vi "prius_ver0.vi"() -> ()   [LabVIEW 2015]
uses:
  <vilib>/Platform/TimedLoop/XDataNode/timing_clust.ctl
  <vilib>/Platform/TimedLoop/XDataNode/nitl_modes.ctl
  <vilib>/Platform/TimedLoop/XDataNode/wakeup.ctl
  <vilib>/myRIO/Instrument Drivers/Onboard IO/DIO/typedefs/DIO Reference.ctl
  <vilib>/myRIO/Common/Instrument Driver Framework/Utilities/typedefs/myRIO Generic Hardware Reference.ctl
  <vilib>/myRIO/Common/Instrument Driver Framework/Utilities/typedefs/Hardware Version Enum.ctl
  <vilib>/myRIO/Common/Instrument Driver Framework/Utilities/typedefs/myRIO v1.0 Reference.ctl
  <vilib>/myRIO/Common/Instrument Driver Framework/Utilities/typedefs/Generic FPGA Reference.ctl
  <vilib>/myRIO/Common/Instrument Driver Framework/myRIO v1.0/DIO/typedefs/DIO Channels List.ctl
  <vilib>/myRIO/Common/Instrument Driver Framework/myRIO v1.0/DIO/typedefs/DIO Channels Enum.ctl
  <vilib>/userdefined/High Color/nirio_resource_hc.ctl
  <vilib>/myRIO/Common/Instrument Driver Framework/myRIO v1.0/DIO/vis/myRIO v1.1 Open DIO.vi
  <vilib>/myRIO/Common/Instrument Driver Framework/Utilities/vis/Validate Channels.vi
  <vilib>/myRIO/Common/Instrument Driver Framework/myRIO v1.0/DIO/vis/myRIO v1.0 Reserve DIO.vi
  <vilib>/myRIO/Instrument Drivers/Onboard IO/PWM/vis/Set Duty Cycle and Frequency.vi
  <vilib>/myRIO/Common/Instrument Driver Framework/myRIO v1.0/DIO/vis/myRIO v1.0 Close DIO.vi
  <vilib>/myRIO/Common/Instrument Driver Framework/myRIO v1.0/AO/vis/myRIO v1.0 Close AO.vi
  <vilib>/myRIO/Common/Instrument Driver Framework/myRIO v1.0/PWM/vis/myRIO v1.0 Close PWM.vi
  <vilib>/myRIO/Common/Instrument Driver Framework/myRIO v1.0/Resource Manager/vis/myRIO v1.0 Reserve Channel List.vi
  <vilib>/myRIO/Common/Instrument Driver Framework/myRIO v1.0/DIO/vis/myRIO v1.0 Build MUX Configuration DIO.vi
  <vilib>/myRIO/Common/Instrument Driver Framework/myRIO v1.0/DIO/vis/myRIO v1.0 Unreserve DIO.vi
  <vilib>/myRIO/Common/Instrument Driver Framework/myRIO v1.0/AO/vis/myRIO v1.0 Unreserve AO.vi
  <vilib>/myRIO/Common/Instrument Driver Framework/myRIO v1.0/PWM/vis/myRIO v1.0 Unreserve PWM.vi
  <vilib>/myRIO/Common/Instrument Driver Framework/myRIO v1.0/Resource Manager/vis/myRIO v1.0 Reserve Channel.vi
  <vilib>/myRIO/Common/Instrument Driver Framework/myRIO v1.0/Resource Manager/vis/myRIO v1.0 Unreserve Channel.vi
  <vilib>/myRIO/Common/Instrument Driver Framework/myRIO v1.0/Resource Manager/vis/myRIO v1.0 Create Configuration List.vi
  <vilib>/myRIO/Common/Instrument Driver Framework/myRIO v1.0/Resource Manager/vis/myRIO v1.0 Unreserve Channel List.vi
  <vilib>/myRIO/Common/Instrument Driver Framework/myRIO v1.0/AO/vis/myRIO v1.0 Build MUX Configuration AO.vi
  <vilib>/myRIO/Common/Instrument Driver Framework/myRIO v1.0/PWM/vis/myRIO v1.0 Build MUX Configuration PWM.vi
  <vilib>/myRIO/Common/Instrument Driver Framework/myRIO v1.0/Resource Manager/vis/myRIO v1.0 Build Mutex Name.vi
  rio_Global.vi
  <vilib>/Utility/error.llb/Error Cluster From Error Code.vi
  <vilib>/myRIO/Common/Instrument Driver Framework/myRIO v1.0/PWM/vis/myRIO v1.0 Write PWM.vi
  <vilib>/Utility/VariantDataType/GetNumericInfo.vi
  <vilib>/myRIO/Common/Instrument Driver Framework/myRIO v1.0/myRIO v1.1 Open.vi
  <vilib>/myRIO/Common/Instrument Driver Framework/Utilities/vis/IO Manager.vi
  <vilib>/myRIO/Common/Instrument Driver Framework/Utilities/vis/Configuration Manager.vi
  <vilib>/myRIO/Common/Instrument Driver Framework/myRIO v1.0/Resource Manager/vis/myRIO v1.0 Configure IO.vi
  <vilib>/myRIO/Common/Instrument Driver Framework/myRIO v1.0/myRIO v1.0 Close.vi
  <vilib>/myRIO/Common/Instrument Driver Framework/myRIO v1.0/DIO/vis/myRIO v1.0 Write DIO.vi
  <vilib>/myRIO/Common/Instrument Driver Framework/myRIO v1.0/AO/vis/myRIO v1.0 Write AO.vi
  <vilib>/myRIO/Common/Instrument Driver Framework/myRIO v1.0/DIO/vis/myRIO v1.0 Shutdown DIO.vi
  <vilib>/myRIO/Common/Instrument Driver Framework/myRIO v1.0/PWM/vis/myRIO v1.0 Shutdown PWM.vi
  <vilib>/Analysis/Matrix/Numeric/Conversions/Array To Matrix - RA2.vi
  <vilib>/Analysis/Matrix/Numeric/Multiply/Multiply - RM,RM.vi
  <vilib>/Analysis/Matrix/Numeric/Add/Add - RM,RM.vi
  <vilib>/Analysis/baseanly.llb/Real Inverse Matrix.vi
  <vilib>/Analysis/Matrix/Numeric/Subtract/Subtract - RM,RM.vi
  <vilib>/Analysis/Matrix/Numeric/Conversions/Array To Matrix - RA.vi
  <vilib>/Analysis/Matrix/Numeric/Multiply/Multiply - R,RM.vi
  <vilib>/Analysis/Matrix/Numeric/Conversions/Matrix To Array - RM.vi
  <vilib>/myRIO/Instrument Drivers/Onboard IO/DIO/vis/myRIO DIO Open.xnode
  <vilib>/platform/TimedLoop/XDataNode/XDataNode.xnode
  <vilib>/myRIO/Instrument Drivers/Onboard IO/DIO/DIO.lvlib
  <vilib>/myRIO/Instrument Drivers/Onboard IO/PWM/PWM.lvlib
  <vilib>/myRIO/Instrument Drivers/Onboard IO/AO/AO.lvlib
  <vilib>/Analysis/Matrix/NI_Matrix.lvlib
  <vilib>/Analysis/NI_AALBase.lvlib
  <vilib>/Platform/TimedLoop/XDataNode/XDNodeRunTimeDep.lvlib
panel:
  in  "Ref_str_torque":dbl
  in  "invgain>1":dbl=4.499999999999998
  in  "mode":bool=TRUE
  in  "x":dbl
  out "Waveform Chart 2":dynamicdata(graph)=[{"t0"=timestamp(3543844041.358625 s since 1904-01-01), "dt"=1.0, "Y"=[0.015263023114702498]}, {"t0"=timestamp(3543844041.358625 s since 1904-01-01), "dt"=1.0, "Y"=[76.5]}]
  in  "x 2":dbl=0.002000000000000001 format="%#_13g"
  out "Ref_VS":dbl
  in  "y":dbl=0.003
  in  "min vel":i32=20
  in  "shift":dbl
  in  "lpf":dbl=0.8 format="%#_13g"
  in  "gain":dbl=0.79
  in  "str_gain":dbl=0.9 format="%#_13g"
  out "handle":dbl=-0.015263023114702498
  out "lane both":bool=TRUE
  out "get map name":bool
  out "map name":T1(ring)=enum."KAIST"
  in  "Steering Control":bool=TRUE
  out "fake_Ref_speed":dbl
  out "fake_Ref_str_ang":dbl
  out "Waveform Chart":dynamicdata(graph)=[{"t0"=timestamp(3543844041.358625 s since 1904-01-01), "dt"=1.0, "Y"=[0.015263023114702498]}, {"t0"=timestamp(3543844041.358625 s since 1904-01-01), "dt"=1.0, "Y"=[76.5]}]
  out "Gear":u8(ring) items=["P", "R", "N", "D"]
  out "read buffer":string="$GNGGA,114428.80,3623.46520,N,12724.00279,E,2,12,0.81,53.9,M,20.0,M,,0000*7B\r\n"
  out "yaw_rate":dbl=0.25
  out "XY Graph":cluster{"Y":dbl[], "Y":dbl[]}[](graph)=[{"Y"=[1.875, 1.875, 1.875, 1.875, 1.875, 1.875, 1.875, 1.875, 1.875, 1.875], "Y"=[0.0, 0.5, 1.0, 1.5, 2.0, 2.5, 3.0, 3.5, 4.0, 4.5]}, {"Y"=[-1.875, -1.875, -1.875, -1.875, -1.875, -1.875, -1.875, -1.875, -1.875, -1.875], "Y"=[0.0, 0.5, 1.0, 1.5, 2.0, 2.5, 3.0, 3.5, 4.0, 4.5]}, {"Y"=[-0.94, 0.94, 0.94, -0.94, -0.94], "Y"=[-3.2, -3.2, 1.5, 1.5, -3.2]}, {"Y"=[0.0, 0.0, 0.0, 0.0, 0.0, 0.0, 0.0, 0.0, 0.0, 0.0], "Y"=[0.0, 0.5, 1.0, 1.5, 2.0, 2.5, 3.0, 3.5, 4.0, 4.5]}, {"Y"=[-0.0, 0.002441079435136828, 0.009765016068527643, 0.021973905883363898, 0.03907124551911778, 0.061061937284492274, 0.08795229619902045, 0.11975005908698932, 0.15646439575426996, 0.19810592228603952, 0.2446867165104507, 0.2962203356814186, 0.3527218364413329, 0.41420779713322275, 0.48069634254055416, 0.5522071711422214, 0.6287615849803672, 0.7103825222489633, 0.7970945927225799, 0.8889241161567654, 0.9858991638044046, 1.0880496032065068, 1.1954071464308669, 1.3080054019486056, 1.4258799303560679, 1.5490683041691753, 1.677610171938241, 1.811547326954198, 1.950923780842551, 2.095785842368791, 2.246182201809347], "Y"=[0.0, 0.5, 1.0, 1.5, 2.0, 2.5, 3.0, 3.5, 4.0, 4.5, 5.0, 5.5, 6.0, 6.5, 7.0, 7.5, 8.0, 8.5, 9.0, 9.5, 10.0, 10.5, 11.0, 11.5, 12.0, 12.5, 13.0, 13.5, 14.0, 14.5, 15.0]}, {"Y"=[-0.0, 0.0008216505896712079, 0.0032866289850517205, 0.00739501506930651, 0.013146941995614725, 0.020542596208514396, 0.029582217474256822, 0.040266098919687465, 0.05259458707971021, 0.06656808195359076, 0.08218703706990027, 0.09945195956012753, 0.11836341024121566, 0.13892200370679575, 0.16112840842706078, 0.18498334685799023, 0.21048759555890229, 0.23764198531947045, 0.2664474012953235, 0.2969047831529963, 0.32901512522389, 0.3627794766672423, 0.39819894164267566, 0.4352746794916982, 0.474007904928726, 0.5143998882415417, 0.5564519555013874, 0.6001654887822383, 0.6455419263903934, 0.6925827631032746, 0.7412895504183155], "Y"=[0.0, 0.5, 1.0, 1.5, 2.0, 2.5, 3.0, 3.5, 4.0, 4.5, 5.0, 5.5, 6.0, 6.5, 7.0, 7.5, 8.0, 8.5, 9.0, 9.5, 10.0, 10.5, 11.0, 11.5, 12.0, 12.5, 13.0, 13.5, 14.0, 14.5, 15.0]}]
  out "Heading":dbl=-179.220077008385
  out "H_GPS":dbl
  out "pos":dbl[](array[numeric])=[1736.3543614568478, 3514.6262112945274]
  in  "GPS init":bool
  out "pos_gps":dbl[](array[numeric])=[42268800.0, 1.0, 1735.3231710957089, 3511.903145121578, -49.202530661854894, 42268800.0, 12.0, 18.0, 0.0, 0.81, 0.81, 0.0, 36.391086666666666, 127.4000465, 73.0] format="%#_19f"
  out "dt":dbl
  out "ecef ref":dbl[](array[numeric])=[-3119987.903302517, 4086549.99824973, 3761829.662354208]
  out "vgain":dbl=1.0353330715599283
  out "vcount":u64=227
  out "hbias":dbl=0.2579217148182668
  out "hcount":u64=1073
  out "get heading":bool
  out "get position":bool=TRUE
  out "heading error":dbl=3.127980429474107
  out "h_gps":dbl
  out "rt":dbl
  out "pos error":dbl=2.9758035193747063
  out "Kalmann init":bool
  out "VS_CAN":dbl
  out "car":refnum<k5>
  out "mdps str_ang":dbl=76.5
  out "eye":refnum<k5>
  out "APV":dbl
  out "PWM GAS":dbl=1000.0 min=1000.0 max=2000.0 step=1.0
  out "Auto":bool
  in  "Steering angle input":dbl(slide) min=-90.0 max=90.0 step=1.0 scale=-90.0..90.0
  in  "Steering angle input":bool=TRUE
  out "T init":i32=20
  out "T out":i32=20
  in  "manual speed":dbl
  in  "Velocity input":bool
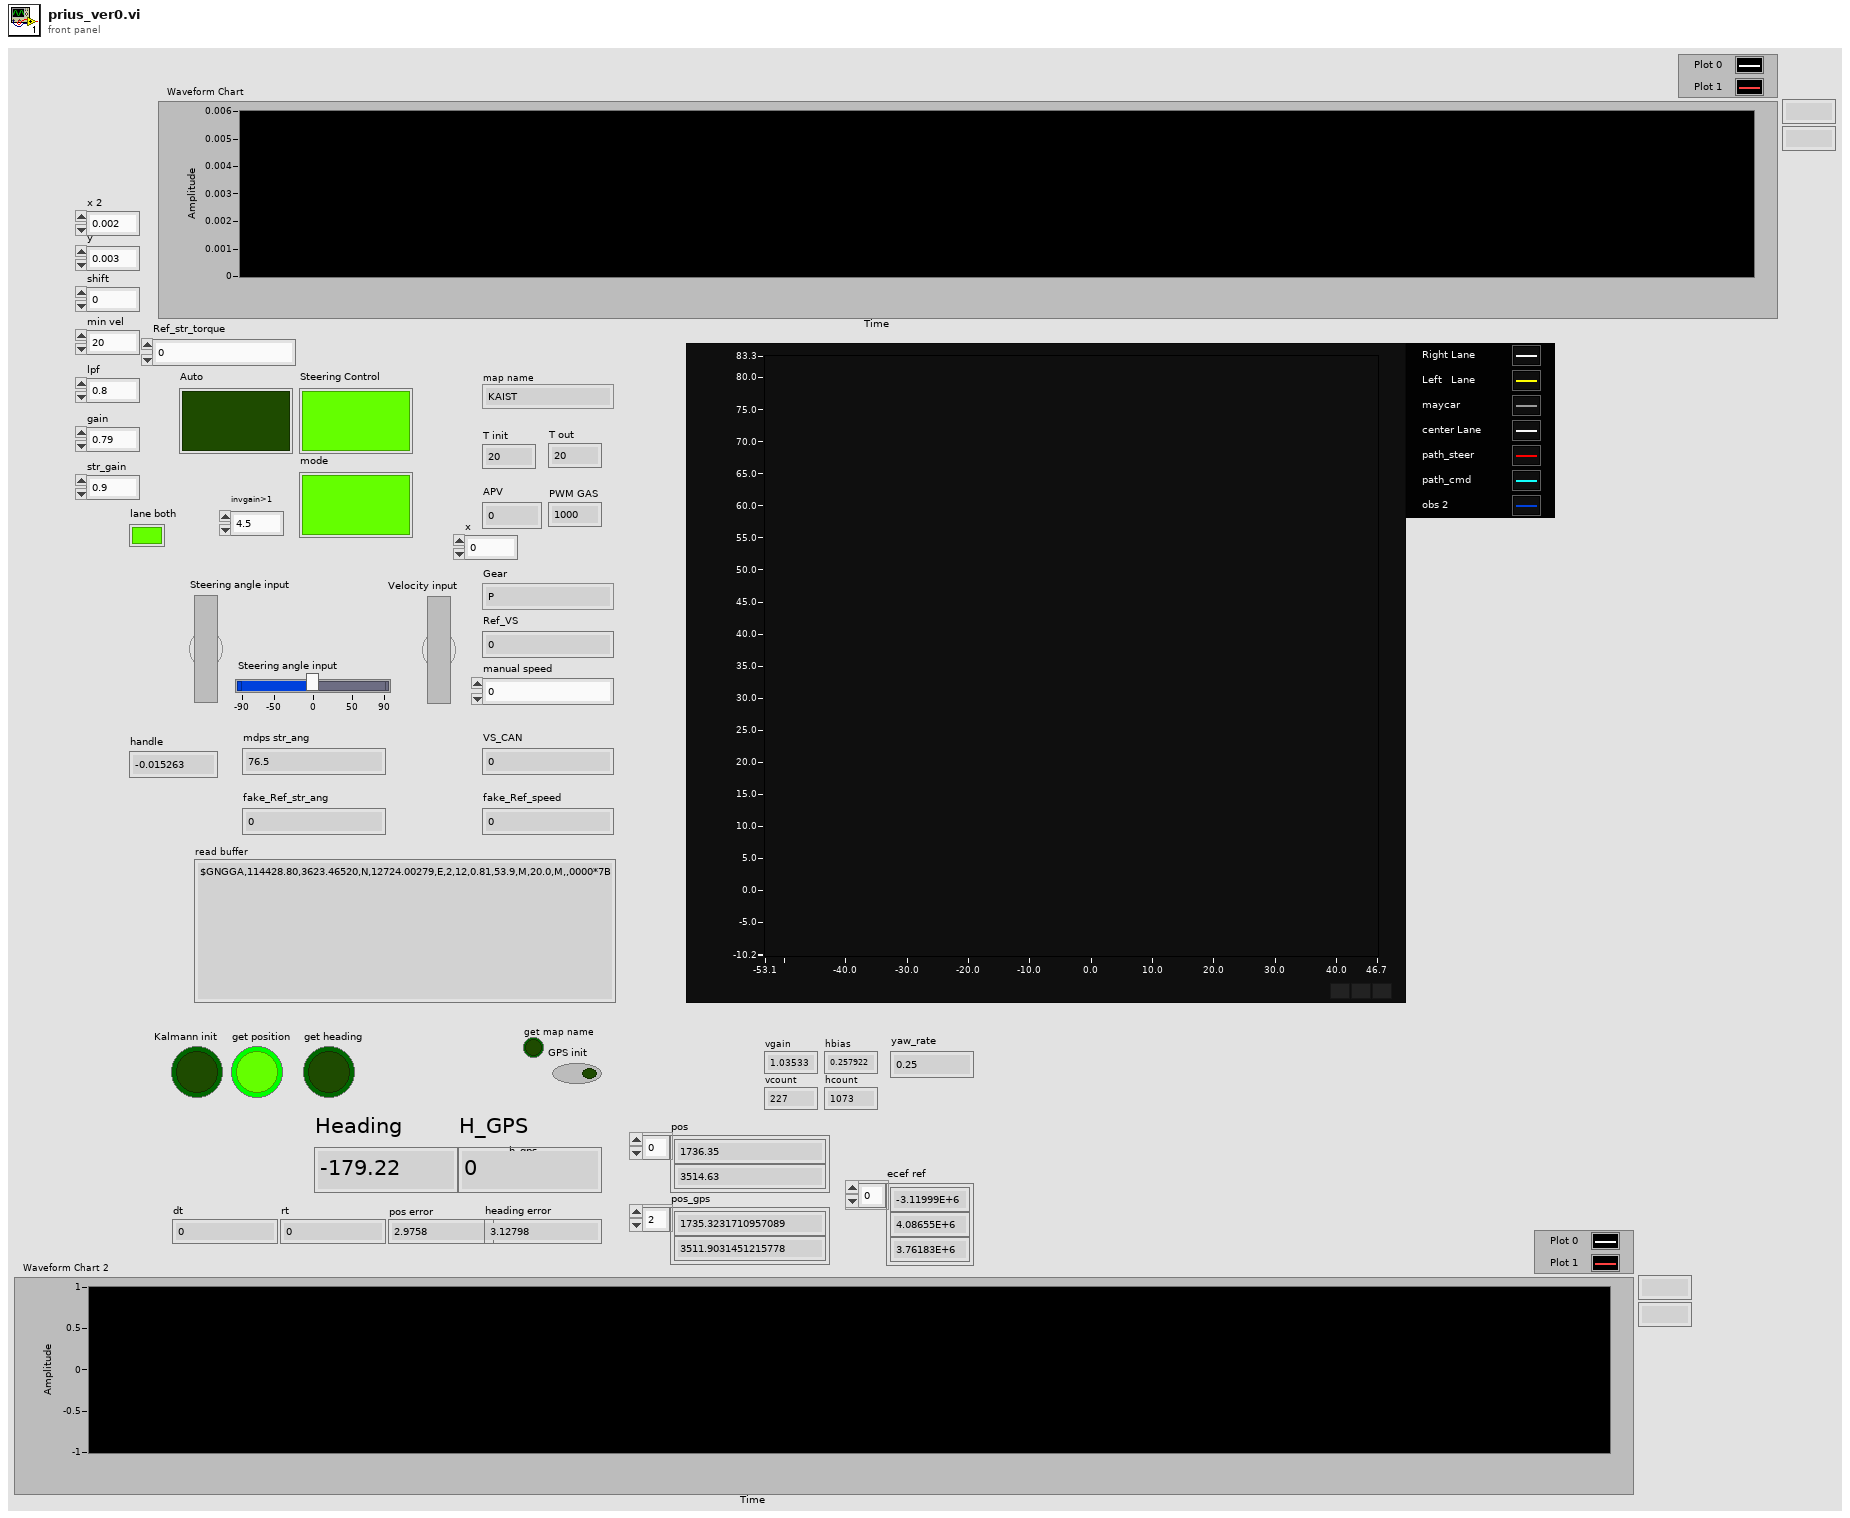
[diagram p1: front panel]
types:
  T1 = enum32{"Namyang", "Hyundai", "KAIST", "Ajou", "Munji", "Airforce", "Car", "KATRI", "Samsung", "Coex", "Gwangnaru"}
  T2 = typedef "XDNodeRunTimeDep.lvlib/timing_clust.ctl" = cluster{"Expected End [f-1]":u64, "Actual End [f-1]":u64, "Finished Late? [f-1]":bool, "Expected End [i-1]":u64, "Actual End [i-1]":u64, "Finished Late? [i-1]":bool, "Expected Start [i]":u64, "Actual Start [i]":u64, "Expected Start [f]":u64, "Actual Start [f]":u64, "Source Name":string, "Structure Name":string, "Period":i64, "Deadline":i64, "Offset":i64, "Start":i64, "Priority":i32, "Timeout":i32, "Mode":T3, "Wakeup Reason":T4, "Error":errorcluster, "Source Type":string, "Secondary Source Type":string, "Global End Time":u64, "Global Start Time":u64, "Frame Duration":u64, "Iteration Duration":u64, "Assigned CPU":i32, "I/O Scan Engine Mode":u32}
  T3 = typedef "XDNodeRunTimeDep.lvlib/nitl_modes.ctl" = enum32{"No Change", "Process missed periods, maintain original phase", "Discard missed periods, maintain original phase", "Process missed periods, ignore original phase", "Discard missed periods, ignore original phase"}
  T4 = typedef "XDNodeRunTimeDep.lvlib/wakeup.ctl" = enum32{"Normal", "Aborted", "Asynchronous wakeup", "Timing source error", "Timed loop error", "Timeout"}
  T5 = typedef "nirio_resource_hc.ctl" = tag
  T6 = typedef "Hardware Version Enum.ctl" = enum16{"Unknown", "myRIO-1900", "myRIO-1950", "roboRIO"}
  T7 = enum16{"Standard", "Buffered", "CRLF", "Immediate"}
  T8 = cluster{"identifier":u32, "timestamp":timestamp, "payload":u8[]}
  T9 = cluster{"connection ID":refnum<k16>, "net address":u32, "port":u16}
  T10 = cluster{"hash":i64, "sys time":i64, "size":i32, "data":u8[]}
  T11 = cluster{"hash":i64, "sys time":i64, "time":dbl, "yaw_rate":dbl, "mdps torque":dbl, "mdps str_ang":dbl, "VS_CAN":dbl, "lat_accel":dbl, "mcp":dbl, "accel pedal value":dbl, "tps":dbl, "odometer":dbl, "battery voltage":dbl, "WHL_SPD_RR":dbl, "WHL_SPD_RL":dbl, "WHL_SPD_FR":dbl, "WHL_SPD_FL":dbl}
  T12 = typedef "PWM.lvlib/PWM Reference.ctl" = cluster{"myRIO Reference":T13, "PWM Channels Enum":T16, "PWM Configuration":T17}
  T13 = typedef "myRIO Generic Hardware Reference.ctl" = cluster{"myRIO Model":T6, "myRIO Hardware Reference":T14}
  T14 = typedef "myRIO v1.0 Reference.ctl" = cluster{"Generic FPGA Reference":T15, "Allow multiple opens":bool}
  T15 = typedef "Generic FPGA Reference.ctl" = refnum<k20>
  T16 = typedef "PWM Channels Enum.ctl" = enum16{"Not Connected", "C/PWM0", "C/PWM1", "A/PWM0", "A/PWM1", "A/PWM2", "B/PWM0", "B/PWM1", "B/PWM2", "PWM/PWM0", "PWM/PWM1", "PWM/PWM2", "PWM/PWM3", "PWM/PWM4", "PWM/PWM5", "PWM/PWM6", "PWM/PWM7", "PWM/PWM8", "PWM/PWM9"}
  T17 = typedef "PWM.lvlib/PWM Configuration.ctl" = cluster{"Frequency":dbl, "Duty Cycle":dbl}
  T18 = typedef "AO.lvlib/AO Reference.ctl" = cluster{"myRIO Reference":T13, "AO Channel List":T19, "AO Scaling Constant List":T21}
  T19 = typedef "AO Channels List.ctl" = T20[]
  T20 = typedef "AO Channels Enum.ctl" = enum16{"Not Connected", "AudioOut/Left", "AudioOut/Right", "C/AO0", "C/AO1", "A/AO0", "A/AO1", "B/AO0", "B/AO1"}
  T21 = typedef "Analog Scaling Constants List.ctl" = T22[]
  T22 = typedef "Analog Scaling Constants.ctl" = cluster{"LSB Weight (Volts)":dbl, "Offset (Volts)":dbl, "Signed?":bool}
  T23 = typedef "DIO.lvlib/DIO Reference.ctl" = cluster{"myRIO Reference":T13, "DIO Channels List":T24}
  T24 = typedef "DIO Channels List.ctl" = T25[]
  T25 = typedef "DIO Channels Enum.ctl" = enum16{"Not Connected", "C/DIO0", "C/DIO1", "C/DIO2", "C/DIO3", "C/DIO4", "C/DIO5", "C/DIO6", "C/DIO7", "A/DIO0", "A/DIO1", "A/DIO2", "A/DIO3", "A/DIO4", "A/DIO5", "A/DIO6", "A/DIO7", "A/DIO8", "A/DIO9", "A/DIO10", "A/DIO11", "A/DIO12", "A/DIO13", "A/DIO14", "A/DIO15", "B/DIO0", "B/DIO1", "B/DIO2", "B/DIO3", "B/DIO4", "B/DIO5", "B/DIO6", "B/DIO7", "B/DIO8", "B/DIO9", "B/DIO10", "B/DIO11", "B/DIO12", "B/DIO13", "B/DIO14", "B/DIO15", "LED0", "LED1", "LED2", "LED3", "Button0", "DIO/DIO0", "DIO/DIO1", "DIO/DIO2", "DIO/DIO3", "DIO/DIO4", "DIO/DIO5", "DIO/DIO6", "DIO/DIO7", "DIO/DIO8", "DIO/DIO9", "SPI/CS0", "SPI/CS1", "SPI/CS2", "SPI/CS3", "LED RADIO (Green)", "LED RADIO (Red)", "LED COMM (Green)", "LED COMM (Red)", "LED MODE (Green)", "LED MODE (Red)"}
  T26 = cluster{"hash":i64, "sys time":i64, "ref_vel":dbl, "ref_steer":dbl, "alert":u8}
  T27 = cluster{"hash":i64, "sys time":i64, "ref_vel":dbl, "ref_steer":dbl}
  T28 = cluster{"hash":i64, "sys time":i64, "Auto":bool, "Run":bool, "Solenoid":bool, "T lim":bool, "brk_enc":u8, "B PWM":u16, "T PWM":u16, "ref_vel":dbl, "ref_bkr_enc":dbl, "ref_apv":dbl, "ref_steer":dbl}
  T29 = typedef "NI_Matrix.lvlib/RealMatrix.ctl" = dbl[][]
  T30 = cluster{"hash":i64, "sys time":i64, "dt":dbl, "x":dbl, "y":dbl, "speed":dbl, "heading":dbl, "yaw_rate":dbl}
  T31 = cluster{"Real 2D Array[0]":dbl, "Real 2D Array[1]":dbl, "Real 2D Array[2]":dbl, "Real 2D Array[3]":dbl, "Real 2D Array[4]":dbl}
  T32 = cluster{"hash":i64, "sys time":i64, "time":dbl, "x":dbl, "y":dbl, "h":dbl, "numSV":i32, "postype":i32, "lag":i32, "hordev":dbl, "lat":dbl, "lon":dbl, "hgt":dbl, "map_idx":i32}
  T33 = cluster{"output[0]":dbl, "output[1]":dbl, "output[2]":dbl, "output[3]":dbl, "output[4]":dbl, "output[5]":dbl, "output[6]":dbl, "output[7]":dbl, "output[8]":dbl, "output[9]":dbl, "output[10]":dbl, "output[11]":dbl, "output[12]":dbl, "output[13]":dbl, "output[14]":dbl}
  T34 = cluster{"hash":i64, "sys time":i64, "time":dbl, "speed":dbl, "heading":dbl, "lat":dbl, "lon":dbl}
  T35 = cluster{"output[0]":dbl, "output[1]":dbl, "output[2]":dbl, "output[3]":dbl, "output[4]":dbl, "output[5]":dbl, "output[6]":dbl}
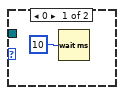
[diagram p2: hidden frame]
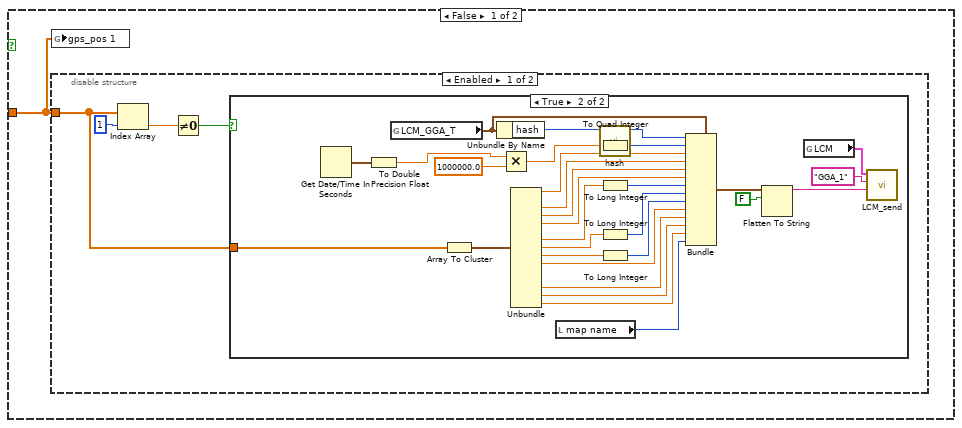
[diagram p4: hidden frame]
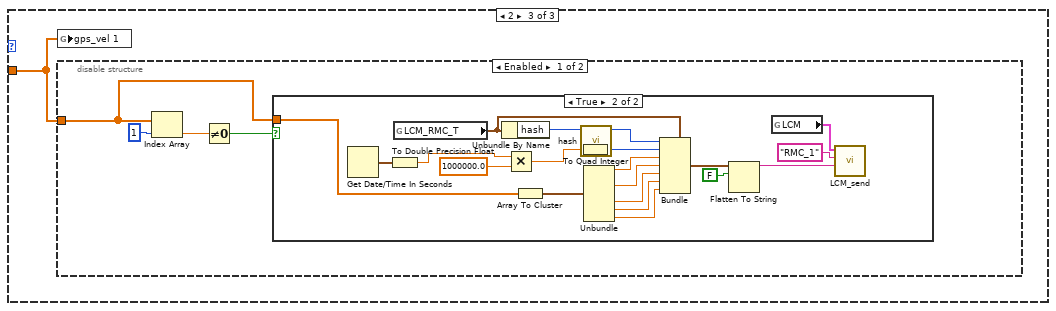
[diagram p7: hidden frame]
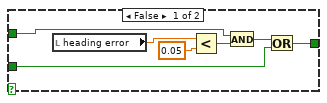
[diagram p13: hidden frame]
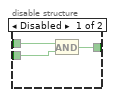
[diagram p14: hidden frame]
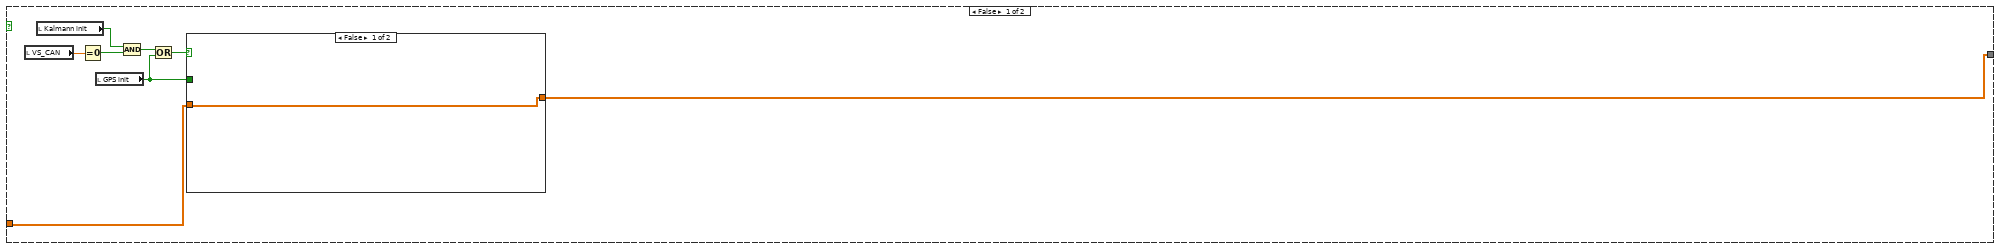
[diagram p15: hidden frame]
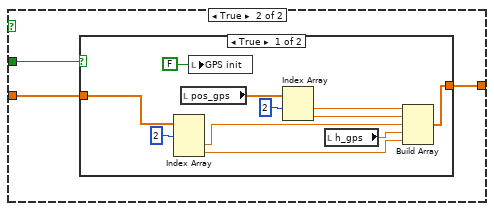
[diagram p16: hidden frame]
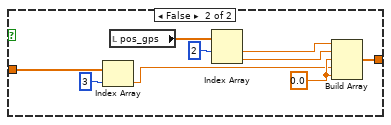
[diagram p17: hidden frame]
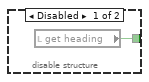
[diagram p19: hidden frame]
diagram:
  n1 = flat-sequence {
    frame #0 {
      w17 = u16 7668 ("port")
      w13 = u16 7665 ("port")
      n2 = disable-structure shown="Enabled" {
        frame Disabled {
        }
        frame Enabled {
          w36 = "Prius" ("Car_name")
          w37 = 0.0 ("Ref_str_ang")
          w38 = 1000.0 ("PWM GAS")
          w34 = FALSE ("Auto SW")
          n3 = global write "rio_Global.vi" "steering torque"(0.0 ("steering")) -> ()
          n4 = global write "rio_Global.vi" "Shift control"(0.0 ("Shift control")) -> ()
          n5 = global write "rio_Global.vi" "Solenoid"(FALSE ("CAN A 1")) -> ()
          n6 = global write "rio_Global.vi" "PWM GAS"(w38) -> ()
          n7 = global write "rio_Global.vi" "PWM Brake"(w38) -> ()
          n8 = global write "rio_Global.vi" "Ref_VS"(w37) -> ()
          n9 = global write "rio_Global.vi" "Ref_str_ang"(w37) -> ()
          n10 = global write "rio_Global.vi" "Auto"(w34) -> ()
          n11 = global write "rio_Global.vi" "Car_name"(w36) -> ()
          n12 = call "car_spec.vi"("Car_name"=w36) -> ("wheel base"=w31:dbl, "ratio"=w32:dbl, "overall width"=w33:dbl)  [unwired: 5 in, 3 out]
          n13 = global write "rio_Global.vi" "Auto SW"(w34) -> ()
          n14 = global write "rio_Global.vi" "ratio"(w32) -> ()
          n15 = global write "rio_Global.vi" "overall width"(w33) -> ()
          n16 = global write "rio_Global.vi" "wheel base"(w31) -> ()
        }
      }
      n17 = local read "eye"() -> (w19:refnum<k5>)
      n18 = local read "car"() -> (w20:refnum<k5>)
      n19 = global read "rio_Global.vi" "LCM PC"() -> (w10:T9)
      n20 = Equal?(x=refnum<k5> refnum ("connection ID"), y=w19) -> (x = y?=w21:bool)
      n21 = Equal?(x=refnum<k5> refnum ("connection ID"), y=w20) -> (x = y?=w23:bool)
      n22 = UDP Open(11:w17) -> (port=w15:refnum<k16>)  [unwired: 4 in, 2 out]
      n23 = Decrement(x=w13) -> (x-1=w12:u16)
      n24 = disable-structure shown="Enabled" {
        disable-tunnel: [w26 w29] -> w14
        disable-tunnel: w12 -> [w25 w30]
        frame Enabled {
          n25 = UDP Open(11:w25) -> (port=w26:refnum<k16>)  [unwired: 4 in, 2 out]
        }
        frame Disabled {
          n26 = String To IP(1:"239.255.76.67" ("name")) -> (0:w27:u32)
          n27 = UDP Multicast Open(10:w27, 11:w30) -> (3:w29:refnum<k16>)  [unwired: 3 in, 2 out]
        }
      }
      n28 = case shown="False" w21 {
        tunnel: w19 -> [w42 _]
        tunnel: [w41 w47] -> w18
        frame False {
          n29 = flat-sequence {
            tunnel: w42 -> [w43]
            tunnel: [w44] -> w41
            frame #0 {
              n30 = TCP Close Connection(connection ID=w43) -> ()  [unwired: 2 in, 2 out]
            }
            frame #1 {
              w45 = u16 3000  # port
              n31 = TCP Open Connection(address="192.168.0.100", remote port or service name=w45) -> (connection ID=w44:refnum<k5>)  [unwired: 3 in, 1 out]
            }
          }
        }
        frame True {
          w48 = u16 3000  # port
          n32 = TCP Open Connection(address="192.168.0.100", remote port or service name=w48) -> (connection ID=w47:refnum<k5>)  [unwired: 3 in, 1 out]
        }
      }
      "eye" <- w18
      n33 = case shown="False" w23 {
        tunnel: w20 -> [w51 _]
        tunnel: [w50 w56] -> w5
        frame False {
          n34 = flat-sequence {
            tunnel: w51 -> [w52]
            tunnel: [w53] -> w50
            frame #0 {
              n35 = TCP Close Connection(connection ID=w52) -> ()  [unwired: 2 in, 2 out]
            }
            frame #1 {
              w54 = u16 4000  # port
              n36 = TCP Open Connection(address="192.168.0.200", remote port or service name=w54) -> (connection ID=w53:refnum<k5>)  [unwired: 3 in, 1 out]
            }
          }
        }
        frame True {
          w57 = u16 4000  # port
          n37 = TCP Open Connection(address="192.168.0.200", remote port or service name=w57) -> (connection ID=w56:refnum<k5>)  [unwired: 3 in, 1 out]
        }
      }
      n38 = Bundle By Name(cluster=w10, "port"=w17, "connection ID"=w15, "net address"=u32 0) -> (w11:T9)
      n39 = global write "rio_Global.vi" "LCM PC"(w11) -> ()
      n40 = String To IP(1:"192.168.0.5" ("name")) -> (0:w2:u32)
      n41 = global read "rio_Global.vi" "LCM"() -> (w9:T9)
      n42 = Bundle By Name(cluster=w9, "port"=w13, "connection ID"=w14, "net address"=w2) -> (w8:T9)
      n43 = global write "rio_Global.vi" "LCM"(w8) -> ()
      n44 = TCP Read(connection ID=w5, bytes to read=999999, 9:1 ("timeout ms (25000)")) -> (connection ID out=→"car":refnum<k5>)  [unwired: 2 in, 2 out]
    }
    frame #1 {
      w87 = tag "B/PWM2"  # Brake
      w101 = tag[] ["B/AO0", "B/AO1"]  # Steering
      w108 = tag[] ["B/DIO4"]  # auto
      w111 = tag "B/PWM0"  # Accel
      w116 = tag[] ["B/DIO5", "B/DIO6"]  # Solenoid
      w78 = tag[] ["C/DIO7", "C/DIO6", "C/DIO5", "C/DIO0"]  # Shift X Eable
      w83 = tag[] ["C/AO0", "C/AO1"]  # Shift
      n45 = local read "eye"() -> (w92:refnum<k5>)
      n46 = local read "car"() -> (w88:refnum<k5>)
      n47 = while {
        tunnel: w92 -> [w302]
        tunnel: [w304] -> w95
        tunnel: [w303] -> w94
        shift-right: [w298] -> _
        shift-left: "" -> [w301]
        stop <- FALSE stop-if-true
        n48 = TCP Read(connection ID=w302, bytes to read=999999, 7:T7."Immediate" ("mode (standard)"), 9:1 ("timeout ms (25000)")) -> (connection ID out=w304:refnum<k5>, data out=w300:string, error out=w303:errorcluster)  [unwired: 1 in]
        n49 = Concatenate Strings(w301, w300) -> (w299:string)
        n50 = case shown="Default" w299 {
          selector: w299 -> [_ w312]
          tunnel: [_ w311] -> w298
          frame "" {
          }
          frame Default {
            n51 = flat-sequence {
              tunnel: w312 -> [w313]
              tunnel: [w314] -> w310
              tunnel: [w313] -> w309
              tunnel: [w343] -> w311
              tunnel: w310 -> [w343]
              tunnel: w309 -> [w342]
              frame #0 {
                n52 = while {
                  shift-right: [w321] -> w314
                  shift-left: w313 -> [w333]
                  stop <- w318 stop-if-true
                  w319 = "S" ("regular expression")
                  n53 = Match Pattern(string=w333, regular expression="S") -> (after substring=w331:string)  [unwired: 1 in, 3 out]
                  n54 = Match Pattern(string=w331, regular expression=" ") -> (before substring=w329:string, after substring=w326:string)  [unwired: 1 in, 2 out]
                  n55 = Hexadecimal String To Number(string=w329) -> (number=w316:u32)  [unwired: 2 in, 1 out]
                  n56 = Match Pattern(string=w326, regular expression=w319) -> (before substring=w325:string, match substring=w320:string, after substring=w322:string)  [unwired: 1 in, 1 out]
                  n57 = Not Equal?(x=w320, y=w319) -> (x != y?=w318:bool)
                  n58 = Concatenate Strings(w320, w322) -> (w321:string)
                  n59 = for {
                    N: 8 -> [_]
                    tunnel: w325 -> [w341]
                    tunnel: [w337] -> w315 mode=indexing
                    i -> [w336]
                    n60 = Multiply(x=2, y=w336) -> (x*y=w339:i32)
                    n61 = String Subset(string=w341, offset (0)=w339, length (rest)=2 ("length (rest)")) -> (substring=w334:string)
                    n62 = Hexadecimal String To Number(string=w334, default (0uL)=u8 0) -> (number=w337:u8)  [unwired: 1 in, 1 out]
                  }
                  n63 = Get Date/Time In Seconds() -> (seconds since 1Jan1904=w324:timestamp)
                  n64 = Bundle By Name(cluster=T8 {"identifier"=0, "timestamp"=timestamp(0 s since 1904-01-01), "payload"=[]} ("can cluster"), "identifier"=w316, "payload"=w315, "timestamp"=w324) -> (w323:T8)
                  n65 = call "mobileye_decoder.vi"("can cluster"=w323, "name"="Mobileye560") -> ()  [unwired: 10 in]
                }
              }
              frame #1 {
                n66 = disable-structure shown="Enabled" {
                  disable-tunnel: w342 -> [w345 _]
                  frame Enabled {
                    n67 = global read "rio_Global.vi" "LCM_CAN_RAW_SNAP"() -> (w358:T10)
                    n68 = Get Date/Time In Seconds() -> (seconds since 1Jan1904=w356:timestamp)
                    n69 = To Double Precision Float(number=w356) -> (double precision float=w355:dbl)
                    n70 = Unbundle By Name(w358) -> ("hash"=w353:i64)
                    n71 = Multiply(x=w355, y=1000000.0) -> (x*y=w357:dbl)
                    n72 = String To Byte Array(string=w345) -> (unsigned byte array=w346:u8[])
                    n73 = To Quad Integer(1:w357) -> (0:w348:i64)
                    n74 = call "hash.vi"("input"=w353) -> ("output"=w359:i64)  [unwired: 10 in]
                    n75 = Array Size(array=w346) -> (size(s)=w347:i32)
                    n76 = Bundle(cluster=w358, "hash"=w359, "sys time"=w348, "size"=w347, "data"=w346) -> (w351:T10)
                    n77 = Flatten To String(anything=w351, prepend array or string size? (T)=FALSE) -> (data string=w349:string)  [unwired: 2 in, 2 out]
                    n78 = global read "rio_Global.vi" "LCM"() -> (w350:T9)
                    n79 = call "LCM_send.vi"("DATA"=w349, "ID"="Mobileye560S", "LCM"=w350) -> ()  [unwired: 7 in, 2 out]
                  }
                  frame Disabled {
                  }
                }
              }
            }
          }
        }
      }
      n80 = while {
        tunnel: w88 -> [w209]
        tunnel: [w211] -> w89
        tunnel: [w210] -> w90
        shift-right: [w205] -> _
        shift-left: "" -> [w208]
        stop <- FALSE stop-if-true
        n81 = TCP Read(connection ID=w209, bytes to read=999999, 7:T7."Immediate" ("mode (standard)"), 9:1 ("timeout ms (25000)")) -> (connection ID out=w211:refnum<k5>, data out=w207:string, error out=w210:errorcluster)  [unwired: 1 in]
        n82 = Concatenate Strings(w208, w207) -> (w206:string)
        n83 = case shown="Default" w206 {
          selector: w206 -> [_ w219]
          tunnel: [_ w220] -> w205
          frame "" {
          }
          frame Default {
            n84 = flat-sequence {
              tunnel: w219 -> [w221]
              tunnel: [w222] -> w218
              tunnel: [w221] -> w217
              tunnel: w218 -> [w251]
              tunnel: w217 -> [w250]
              tunnel: [w251] -> w216
              tunnel: [w297] -> w220
              tunnel: w216 -> [w297]
              frame #0 {
                n85 = while {
                  shift-right: [w231] -> w222
                  shift-left: w221 -> [w241]
                  stop <- w228 stop-if-true
                  w229 = "S" ("regular expression")
                  n86 = Match Pattern(string=w241, regular expression="S") -> (after substring=w239:string)  [unwired: 1 in, 3 out]
                  n87 = Match Pattern(string=w239, regular expression=" ") -> (before substring=w237:string, after substring=w235:string)  [unwired: 1 in, 2 out]
                  n88 = Hexadecimal String To Number(string=w237) -> (number=w226:u32)  [unwired: 2 in, 1 out]
                  n89 = Match Pattern(string=w235, regular expression=w229) -> (before substring=w234:string, match substring=w230:string, after substring=w232:string)  [unwired: 1 in, 1 out]
                  n90 = Not Equal?(x=w230, y=w229) -> (x != y?=w228:bool)
                  n91 = Concatenate Strings(w230, w232) -> (w231:string)
                  n92 = for {
                    N: 8 -> [_]
                    tunnel: w234 -> [w249]
                    tunnel: [w245] -> w225 mode=indexing
                    i -> [w244]
                    n93 = Multiply(x=2, y=w244) -> (x*y=w247:i32)
                    n94 = String Subset(string=w249, offset (0)=w247, length (rest)=2 ("length (rest)")) -> (substring=w242:string)
                    n95 = Hexadecimal String To Number(string=w242, default (0uL)=u8 0) -> (number=w245:u8)  [unwired: 1 in, 1 out]
                  }
                  n96 = Get Date/Time In Seconds() -> (seconds since 1Jan1904=w233:timestamp)
                  n97 = Bundle By Name(cluster=T8 {"identifier"=0, "timestamp"=timestamp(0 s since 1904-01-01), "payload"=[]} ("can cluster"), "identifier"=w226, "payload"=w225, "timestamp"=w233) -> (w223:T8)
                  n98 = global read "rio_Global.vi" "Car_name"() -> (w224:string)
                  n99 = call "can decoder.vi"("can cluster"=w223, "name"=w224) -> ()  [unwired: 10 in]
                }
              }
              frame #1 {
                n100 = disable-structure shown="Enabled" {
                  disable-tunnel: w250 -> [w252 _]
                  frame Enabled {
                    n101 = global read "rio_Global.vi" "LCM_CAN_RAW_SNAP"() -> (w254:T10)
                    n102 = Get Date/Time In Seconds() -> (seconds since 1Jan1904=w256:timestamp)
                    n103 = To Double Precision Float(number=w256) -> (double precision float=w257:dbl)
                    n104 = Unbundle By Name(w254) -> ("hash"=w259:i64)
                    n105 = Multiply(x=w257, y=1000000.0) -> (x*y=w255:dbl)
                    n106 = String To Byte Array(string=w252) -> (unsigned byte array=w267:u8[])
                    n107 = To Quad Integer(1:w255) -> (0:w265:i64)
                    n108 = call "hash.vi"("input"=w259) -> ("output"=w253:i64)  [unwired: 10 in]
                    n109 = Array Size(array=w267) -> (size(s)=w266:i32)
                    n110 = Bundle(cluster=w254, "hash"=w253, "sys time"=w265, "size"=w266, "data"=w267) -> (w261:T10)
                    n111 = global read "rio_Global.vi" "Car_name"() -> (w264:string)
                    n112 = Flatten To String(anything=w261, prepend array or string size? (T)=FALSE) -> (data string=w263:string)  [unwired: 2 in, 2 out]
                    n113 = global read "rio_Global.vi" "LCM"() -> (w262:T9)
                    n114 = call "LCM_send.vi"("DATA"=w263, "ID"=w264, "LCM"=w262) -> ()  [unwired: 7 in, 2 out]
                  }
                  frame Disabled {
                  }
                }
              }
              frame #2 {
                n115 = Get Date/Time In Seconds() -> (seconds since 1Jan1904=w288:timestamp)
                n116 = global read "rio_Global.vi" "LCM_CAN_T"() -> (w270:T11)
                n117 = To Double Precision Float(number=w288) -> (double precision float=w289:dbl)
                n118 = global read "rio_Global.vi" "C_mdps str_ang"() -> (w269:dbl)
                n119 = global read "rio_Global.vi" "C_battery voltage"() -> (w273:dbl)
                n120 = global read "rio_Global.vi" "C_WHL_SPD_RR"() -> (w274:dbl)
                n121 = global read "rio_Global.vi" "C_WHL_SPD_RL"() -> (w275:dbl)
                n122 = global read "rio_Global.vi" "C_WHL_SPD_FR"() -> (w271:dbl)
                n123 = global read "rio_Global.vi" "C_WHL_SPD_FL"() -> (w276:dbl)
                n124 = global read "rio_Global.vi" "C_mdps torque"() -> (w283:dbl)
                n125 = Unbundle By Name(w270) -> ("hash"=w291:i64)
                n126 = Multiply(x=w289, y=1000000.0) -> (x*y=w287:dbl)
                n127 = global read "rio_Global.vi" "C_odometer"() -> (w277:dbl)
                n128 = global read "rio_Global.vi" "C_yaw_rate"() -> (w284:dbl)
                n129 = global read "rio_Global.vi" "C_VS_CAN"() -> (w282:dbl)
                n130 = global read "rio_Global.vi" "C_MCP"() -> (w280:dbl)
                n131 = global read "rio_Global.vi" "C_APV"() -> (w279:dbl)
                n132 = To Quad Integer(1:w287) -> (0:w296:i64)
                n133 = Negate(x=w269) -> (-x=w268:dbl)
                n134 = call "hash.vi"("input"=w291) -> ("output"=w286:i64)  [unwired: 10 in]
                n135 = global read "rio_Global.vi" "time"() -> (w285:dbl)
                n136 = Bundle(cluster=w270, "hash"=w286, "sys time"=w296, "time"=w285, "yaw_rate"=w284, "mdps torque"=w283, "mdps str_ang"=w268, "VS_CAN"=w282, "lat_accel"=0.0, "mcp"=w280, "accel pedal value"=w279, "tps"=0.0, "odometer"=w277, "battery voltage"=w273, "WHL_SPD_RR"=w274, "WHL_SPD_RL"=w275, "WHL_SPD_FR"=w271, "WHL_SPD_FL"=w276) -> (w293:T11)
                n137 = Flatten To String(anything=w293, prepend array or string size? (T)=FALSE) -> (data string=w295:string)  [unwired: 2 in, 2 out]
                n138 = global read "rio_Global.vi" "LCM"() -> (w294:T9)
                n139 = call "LCM_send.vi"("DATA"=w295, "ID"="CAN_T", "LCM"=w294) -> ()  [unwired: 7 in, 2 out]
              }
            }
          }
        }
      }
      n140 = call <vilib>:"Smart Open.vi"("Allow multiple opens?"=FALSE, "Channel Name"=w87) -> ("error out"=w61:errorcluster, "PWM Ref Out"=w64:T12)  [unwired: 8 in]
      n141 = call <vilib>:"Smart Open.vi"("Allow multiple opens?"=FALSE, "Channel Name"=w111) -> ("error out"=w69:errorcluster, "PWM Ref Out"=w68:T12)  [unwired: 8 in]
      n142 = call <vilib>:"Set Frequency.vi"("error in (no error)"=w61, "Frequency [Hz]"=50.0, "PWM Ref In"=w64) -> ("error out"=w60:errorcluster, "PWM Ref Out"=w63:T12)  [unwired: 6 in]
      n143 = call <vilib>:"Set Frequency.vi"("error in (no error)"=w69, "Frequency [Hz]"=50.0, "PWM Ref In"=w68) -> ("error out"=w66:errorcluster, "PWM Ref Out"=w67:T12)  [unwired: 6 in]
      n144 = call <vilib>:"Smart Open.vi"("Allow multiple opens?"=TRUE, "Channel Names"=w101) -> ("error out"=w99:errorcluster, "AO Ref Out"=w100:T18)  [unwired: 8 in]
      n145 = call <vilib>:"Smart Open.vi"("Allow multiple opens?"=FALSE, "Channel Names"=w108) -> ("error out"=w106:errorcluster, "DIO Ref Out"=w107:T23)  [unwired: 8 in]
      n146 = xnode "myRIO DIO Open.xnode"("Allow multiple opens?"=TRUE, "Channel Names"=w116) -> ("error out"=w114:errorcluster, "DIO Ref Out"=w115:T23)  [unwired: 1 in]
      n147 = xnode "myRIO DIO Open.xnode"("Allow multiple opens?"=TRUE, "Channel Names"=w78) -> ("error out"=w73:errorcluster, "DIO Ref Out"=w76:T23)  [unwired: 1 in]
      n148 = call <vilib>:"Smart Open.vi"("Allow multiple opens?"=TRUE, "Channel Names"=w83) -> ("error out"=w79:errorcluster, "AO Ref Out"=w82:T18)  [unwired: 8 in]
      n149 = node-c288(i64 10 ("Period")) -> (w72:T2)  [unwired: 3 in]
      n150 = timed-loop {
        tunnel: w115 -> [w181]
        tunnel: [w182] -> w113
        tunnel: w114 -> [w180]
        tunnel: [w176] -> w112
        tunnel: w107 -> [w174]
        tunnel: [w174] -> w105
        tunnel: w106 -> [w173]
        tunnel: [w173] -> w104
        tunnel: w100 -> [w172]
        tunnel: [w170] -> w98
        tunnel: w99 -> [w171]
        tunnel: [w169] -> w97
        tunnel: w67 -> [w178]
        tunnel: [w179] -> w110
        tunnel: w66 -> [w177]
        tunnel: [w175] -> w109
        tunnel: w63 -> [w167]
        tunnel: [w166] -> w85
        tunnel: w82 -> [w165]
        tunnel: [w164] -> w81
        tunnel: [w163] -> w80
        tunnel: w79 -> [w162]
        tunnel: w76 -> [w161]
        tunnel: [w160] -> w75
        tunnel: [w159] -> w74
        tunnel: w73 -> [w158]
        timing: w72 -> [_]
        timing-out: [_] -> w71
        tunnel: w60 -> [w128]
        tunnel: [w127] -> w59
        stop <- FALSE ("Auto") stop-if-true
        w148 = 0.0 ("y")
        n151 = node-c288() -> ()  [unwired: 1 in]
        n152 = global read "rio_Global.vi" "PWM Brake"() -> (w120:dbl)
        n153 = global read "rio_Global.vi" "PWM GAS"() -> (w123:dbl)
        n154 = global read "rio_Global.vi" "Solenoid"() -> (w121:bool)
        n155 = global read "rio_Global.vi" "steering torque"() -> (w144:dbl)
        n156 = global read "rio_Global.vi" "Shift control"() -> (w132:dbl)
        n157 = global read "rio_Global.vi" "C_VS_CAN"() -> (w140:dbl)
        n158 = global read "rio_Global.vi" "Auto"() -> (w119:bool)
        n159 = global read "rio_Global.vi" "Auto"() -> (w124:bool)
        n160 = global read "rio_Global.vi" "Auto"() -> (w122:bool)
        n161 = Select(t=w121, s=w122, f=w122) -> (s? t:f=w126:bool)
        n162 = Negate(x=w144) -> (-x=w146:dbl)
        n163 = Equal To 0?(x=w140) -> (x = 0?=w130:bool)
        n164 = Not Equal To 0?(x=w132) -> (x != 0?=w131:bool)
        n165 = Select(t=w120, s=w119, f=1000.0) -> (s? t:f=w142:dbl)
        n166 = Select(t=w123, s=w124, f=1000.0) -> (s? t:f=w147:dbl)
        n167 = global read "rio_Global.vi" "Auto"() -> (w145:bool)
        n168 = global read "rio_Global.vi" "Auto"() -> (w141:bool)
        n169 = Build Array(w126, w126) -> (w152:bool[])
        n170 = Select(t=w146, s=w145, f=w148) -> (s? t:f=w149:dbl)
        n171 = call <vilib>:"Write.vi"("error in (no error)"=w180, "Values"=w152, "DIO Ref In"=w181) -> ("error out"=w176:errorcluster, "DIO Ref Out"=w182:T23)  [unwired: 6 in]
        n172 = Compound Arithmetic op=AND(w130, w141, w131) -> (w137:bool)
        n173 = Divide(x=w142, y=20000.0) -> (x/y=w129:dbl)
        n174 = Divide(x=w147, y=20000.0) -> (x/y=w150:dbl)
        n175 = Max & Min(x=w149, y=w148) -> (min(x,y)=w154:dbl)  [unwired: 1 out]
        n176 = Select(t=w132, s=w137, f=0.0 ("element")) -> (s? t:f=w134:dbl)
        n177 = Build Array(w137, w137, w137, FALSE ("element")) -> (w139:bool[])
        n178 = call <vilib>:"Write.vi"("error in (no error)"=w158, "Values"=w139, "DIO Ref In"=w161) -> ("error out"=w159:errorcluster, "DIO Ref Out"=w160:T23)  [unwired: 6 in]
        n179 = Negate(x=w154) -> (-x=w153:dbl)
        n180 = call <vilib>:"Set Duty Cycle.vi"("error in (no error)"=w128, "Duty Cycle"=w129, "PWM Ref In"=w167) -> ("error out"=w127:errorcluster, "PWM Ref Out"=w166:T12)  [unwired: 6 in]
        n181 = call <vilib>:"Set Duty Cycle.vi"("error in (no error)"=w177, "Duty Cycle"=w150, "PWM Ref In"=w178) -> ("error out"=w175:errorcluster, "PWM Ref Out"=w179:T12)  [unwired: 6 in]
        n182 = Max & Min(x=0.0, y=w149) -> (max(x,y)=w155:dbl)  [unwired: 1 out]
        n183 = Build Array(0.0 ("element"), w134) -> (w133:dbl[])
        n184 = call <vilib>:"Write.vi"("error in (no error)"=w162, "Values"=w133, "AO Ref In"=w165) -> ("error out"=w163:errorcluster, "AO Ref Out"=w164:T18)  [unwired: 6 in]
        n185 = Build Array(w155, w153) -> (w157:dbl[])
        n186 = call <vilib>:"Write.vi"("error in (no error)"=w171, "Values"=w157, "AO Ref In"=w172) -> ("error out"=w169:errorcluster, "AO Ref Out"=w170:T18)  [unwired: 6 in]
        n187 = node-c288() -> ()  [unwired: 1 out]
      }
      n188 = node-c288(w71) -> ()  [unwired: 1 out]
      n189 = call <vilib>:"Close.vi"("error in (no error)"=w97, "AO Ref In"=w98) -> ()  [unwired: 9 in, 1 out]
      n190 = call <vilib>:"Close.vi"("error in (no error)"=w59, "PWM Ref In"=w85) -> ()  [unwired: 9 in, 1 out]
      n191 = call <vilib>:"Close.vi"("error in (no error)"=w104, "DIO Ref In"=w105) -> ()  [unwired: 9 in, 1 out]
      n192 = call <vilib>:"Close.vi"("error in (no error)"=w109, "PWM Ref In"=w110) -> ()  [unwired: 9 in, 1 out]
      n193 = call <vilib>:"Close.vi"("error in (no error)"=w112, "DIO Ref In"=w113) -> ()  [unwired: 9 in, 1 out]
      n194 = call <vilib>:"Close.vi"("error in (no error)"=w74, "DIO Ref In"=w75) -> ()  [unwired: 9 in, 1 out]
      n195 = call <vilib>:"Close.vi"("error in (no error)"=w80, "AO Ref In"=w81) -> ()  [unwired: 9 in, 1 out]
      n196 = TCP Close Connection(connection ID=w95, error in (no error)=w94) -> ()  [unwired: 1 in, 2 out]
      n197 = TCP Close Connection(connection ID=w89, error in (no error)=w90) -> ()  [unwired: 1 in, 2 out]
    }
  }
  n198 = flat-sequence {
    frame #0 {
      w380 = 0.0 ("fake_Ref_str_ang")
      w379 = FALSE ("Velocity input")
      n199 = local write "manual speed"(0.0 ("manual speed")) -> ()
      n200 = local write "Steering angle input"(0.0 ("con_vs")) -> ()
      n201 = local write "mode"(FALSE ("mode")) -> ()
      n202 = local write "Steering angle input"(FALSE ("Steering torque input")) -> ()
      n203 = global write "rio_Global.vi" "lane width"(3.5 ("lane width")) -> ()
      n204 = local write "Velocity input"(w379) -> ()
      n205 = local write "Steering Control"(w379) -> ()
      "fake_Ref_str_ang" <- w380
      "fake_Ref_speed" <- w380
      "lane both" <- FALSE ("lane both")
    }
    frame #1 {
      n206 = while {
        stop <- FALSE stop-if-true
        n207 = flat-sequence {
          tunnel: [w697] -> w384
          tunnel: w384 -> [w721]
          frame #0 {
            n208 = Wait Until Next ms Multiple(millisecond multiple=u32 10) -> ()  [unwired: 1 out]
          }
          frame #1 {
            n209 = disable-structure shown="Enabled" {
              disable-tunnel: [w390 _] -> w388
              disable-tunnel: [w389 _] -> w387
              frame Disabled {
                n210 = global read "rio_Global.vi" "LCM PC"() -> (w391:T9)
                n211 = call "LCM_read.vi"("LCM"=w391) -> ("data"=w389:string, "ID"=w390:string)  [unwired: 7 in, 2 out]
              }
              frame Enabled {
              }
            }
            n212 = case shown="Default" w388 {
              tunnel: w387 -> [_ w676]
              frame Default {
                n213 = flat-sequence {
                  frame #0 {
                    w410 = 2 ("index")
                    w414 = 2 ("index")
                    n214 = global read "rio_Global.vi" "C_VS_CAN"() -> (w399:dbl)
                    n215 = global read "rio_Global.vi" "M_lane_right"() -> (w407:dbl[])
                    n216 = global read "rio_Global.vi" "M_headway"() -> (w393:dbl)
                    n217 = global read "rio_Global.vi" "M_lane_left"() -> (w406:dbl[])
                    n218 = Divide(x=w399, y=3.6) -> (x/y=w397:dbl)
                    n219 = Multiply(x=w397, y=w393) -> (x*y=w396:dbl)
                    n220 = Index Array(array=w406, index=w414) -> (element=w413:dbl)
                    n221 = Index Array(array=w407, index=w410) -> (element=w411:dbl)
                    n222 = Greater Or Equal?(x=w413, y=w414) -> (x >= y?=w412:bool)
                    n223 = Greater Or Equal?(x=w411, y=w410) -> (x >= y?=w409:bool)
                    n224 = Multiply(x=w396, y=2.0) -> (x*y=w395:dbl)
                    n225 = local read "lane both"() -> (w417:bool)
                    n226 = Or(x=w412, y=w409) -> (x .or. y?=w418:bool)
                    n227 = And(x=w412, y=w409) -> (x .and. y?=w416:bool)
                    n228 = Not Equal To 0?(x=w393) -> (x != 0?=w392:bool)
                    n229 = And(x=w418, y=w417) -> (x .and. y?=w415:bool)
                    n230 = Max & Min(x="x", y=w395) -> (min(x,y)=w400:dbl)  [unwired: 1 out]
                    n231 = case shown="True" w392 {
                      tunnel: w400 -> [_ w421]
                      frame False {
                      }
                      frame True {
                        n232 = global write "rio_Global.vi" "Ref_VS"(w421) -> ()
                      }
                    }
                    n233 = Or(x=w416, y=w415) -> (x .or. y?=w408:bool)
                    n234 = case shown="True" w408 {
                      tunnel: w406 -> [_ w425]
                      tunnel: w407 -> [_ w423]
                      tunnel: [_ w429] -> w419
                      frame False {
                        n235 = local write "lane both"(FALSE ("lane both")) -> ()
                      }
                      frame True {
                        w427 = 2 ("index")
                        w432 = 2 ("index")
                        n236 = Index Array(array=w425, index=w432) -> (element=w431:dbl)
                        n237 = Index Array(array=w423, index=w427) -> (element=w428:dbl)
                        n238 = Greater Or Equal?(x=w428, y=w427) -> (x >= y?=w424:bool)
                        n239 = Greater Or Equal?(x=w431, y=w432) -> (x >= y?=w426:bool)
                        n240 = And(x=w426, y=w424) -> (x .and. y?=w430:bool)
                        n241 = case shown="False" w430 {
                          tunnel: w425 -> [w454 w456]
                          tunnel: w423 -> [w449 w455]
                          tunnel: [w447 w463] -> w429
                          tunnel: w426 -> [w433 _]
                          frame False {
                            w442 = 0.2 ("y")
                            w445 = 5 ("index")
                            w453 = 5 ("index")
                            n242 = global read "rio_Global.vi" "overall width"() -> (w435:dbl)
                            n243 = Index Array(array=w454, index=w453) -> (element=w451:dbl)
                            n244 = Index Array(array=w449, index=w445) -> (element=w444:dbl)
                            n245 = global read "rio_Global.vi" "lane width"() -> (w434:dbl)
                            n246 = Multiply(x=w435, y=w442) -> (x*y=w440:dbl)
                            n247 = Add(x=w440, y=w442) -> (x+y=w436:dbl)
                            n248 = Add(x=1.0 ("y"), y=w440) -> (x+y=w437:dbl)
                            n249 = Multiply(x=w434, y=0.5) -> (x*y=w439:dbl)
                            n250 = In Range and Coerce(upper limit=w437, x=w439, lower limit=w436) -> (coerced(x)=w438:dbl)  [unwired: 1 out]
                            n251 = Add(x=w451, y=w438) -> (x+y=w450:dbl)
                            n252 = Subtract(x=w444, y=w438) -> (x-y=w443:dbl)
                            n253 = Replace Array Subset(array=w454, new element=w450, index=w453) -> (w448:dbl[])
                            n254 = Replace Array Subset(array=w449, new element=w443, index=w445) -> (w446:dbl[])
                            n255 = Select(t=w448, s=w433, f=w446) -> (s? t:f=w447:dbl[])
                          }
                          frame True {
                            n256 = Add(x=w456, y=w455) -> (x+y=w465:dbl[])
                            n257 = Index Array(array=w455, index=5) -> (element=w461:dbl)
                            n258 = Index Array(array=w456, index=5) -> (element=w458:dbl)
                            n259 = local write "lane both"(TRUE ("lane both")) -> ()
                            n260 = Subtract(x=w461, y=w458) -> (x-y=w457:dbl)
                            n261 = global write "rio_Global.vi" "lane width"(w457) -> ()
                            n262 = Multiply(x=0.5, y=w465) -> (x*y=w463:dbl[])
                          }
                        }
                      }
                    }
                    n263 = Empty Array?(array=w419) -> (empty?=w420:bool)
                    n264 = global write "rio_Global.vi" "M_lane_center"(w419) -> ()
                    n265 = case shown="False" w420 {
                      tunnel: w419 -> [w474 _]
                      tunnel: [w466 w583] -> w405
                      frame False {
                        n266 = global read "rio_Global.vi" "x_view 2"() -> (w473:dbl[])
                        n267 = disable-structure shown="Enabled" {
                          disable-tunnel: w474 -> [w496 _]
                          disable-tunnel: w473 -> [w495 w505]
                          disable-tunnel: [w494 w505] -> w471
                          frame Disabled {
                            n268 = Index Array(array=w496, index=10) -> (element=w501:dbl)
                            n269 = Multiply(x=w501, y=2.0) -> (x*y=w503:dbl)
                            n270 = Round Toward -Infinity(1:w503) -> (0:w498:dbl)
                            n271 = Max & Min(x=10.0, y=w498) -> (max(x,y)=w504:dbl)  [unwired: 1 out]
                            n272 = Array Subset(array=w495, index=0, length=w504) -> (w494:dbl[])
                          }
                          frame Enabled {
                          }
                        }
                        n273 = global read "rio_Global.vi" "C_VS_CAN"() -> (w470:dbl)
                        n274 = disable-structure shown="Enabled" {
                          disable-tunnel: w470 -> [w492 w493]
                          disable-tunnel: [w487 w493] -> w469
                          frame Disabled {
                            w488 = 32.0  # old 42
                            w489 = 15.0  # old 9
                            n275 = Subtract(x=w492, y=10.0) -> (x-y=w490:dbl)
                            n276 = In Range and Coerce(upper limit=w488, x=w490, lower limit=w489) -> (coerced(x)=w487:dbl)  [unwired: 1 out]
                          }
                          frame Enabled {
                          }
                        }
                        n277 = Index Array(array=w474, index #1=7 ("index"), index #2=6 ("index"), index #3=9 ("index"), index #4=5 ("index")) -> (element #1=w475:dbl, element #2=w482:dbl, element #3=w480:dbl, element #4=w486:dbl)
                        n278 = Square(x=w471) -> (x^2=w476:dbl[])
                        n279 = Compound Arithmetic op=MULTIPLY(w475, w471, w476) -> (w479:dbl[])
                        n280 = Compound Arithmetic op=MULTIPLY(w476, w482) -> (w478:dbl[])
                        n281 = Compound Arithmetic op=MULTIPLY(w471, w480) -> (w477:dbl[])
                        n282 = Compound Arithmetic op=ADD(w479, w478, w477, w486) -> (w472:dbl[])
                        n283 = Multiply(x=w469, y=2.0 ("y 2")) -> (x*y=w468:dbl)
                        n284 = flat-sequence {
                          tunnel: w468 -> [w526]
                          tunnel: w471 -> [w525]
                          tunnel: w472 -> [w517]
                          tunnel: [w510] -> w466
                          frame #0 {
                            n285 = disable-structure shown="Enabled" {
                              disable-tunnel: w526 -> [w544 w554]
                              disable-tunnel: w525 -> [w543 w556]
                              disable-tunnel: [w542 w559] -> w521
                              disable-tunnel: w517 -> [w532 w558]
                              frame Disabled {
                                n286 = Interpolate 1D Array(1:w544, 2:w543) -> (0:w545:dbl)
                                n287 = Interpolate 1D Array(1:w544, 2:w532) -> (0:w546:dbl)
                                n288 = Square(x=w546) -> (x^2=w535:dbl)
                                n289 = Square(x=w545) -> (x^2=w536:dbl)
                                n290 = Absolute Value(x=w546) -> (abs(x)=w534:dbl)
                                n291 = Greater Or Equal?(x=w534, y=w545) -> (x >= y?=w533:bool)
                                n292 = Add(x=w535, y=w536) -> (x+y=w537:dbl)
                                n293 = Divide(x=w537, y=w546) -> (x/y=w538:dbl)
                                n294 = Multiply(x=w538, y=0.5) -> (x*y=w540:dbl)
                                n295 = Select(t=w546, s=w533, f=w540) -> (s? t:f=w527:dbl)
                                n296 = Not A Number/Path/Refnum?(number/path/refnum=w527) -> (NaN/Path/Refnum?=w530:bool)
                                n297 = global read "rio_Global.vi" "wheel base"() -> (w531:dbl)
                                n298 = Select(t=inf, s=w530, f=w527) -> (s? t:f=w528:dbl)
                                n299 = Divide(x=w531, y=w528) -> (x/y=w541:dbl)
                                n300 = Inverse Tangent(1:w541) -> (0:w542:dbl)
                              }
                              frame Enabled {
                                n301 = Subtract(x=w554, y="min vel") -> (x-y=w552:dbl)
                                n302 = Array Subset(array=w558, index="min vel") -> (w557:dbl[])  [unwired: 1 in]
                                n303 = Array Subset(array=w556, index="min vel") -> (w555:dbl[])  [unwired: 1 in]
                                n304 = Round Toward -Infinity(1:w552) -> (0:w551:dbl)
                                n305 = Max & Min(x=1.0, y=w551) -> (max(x,y)=w550:dbl)  [unwired: 1 out]
                                n306 = for {
                                N: w550 -> [_]
                                tunnel: w555 -> [w566] mode=indexing
                                tunnel: w557 -> [w567] mode=indexing
                                tunnel: [w565] -> w548 mode=indexing
                                tunnel: [w564] -> w562 mode=indexing
                                i -> [w565]
                                n307 = Square(x=w567) -> (x^2=w575:dbl)
                                n308 = Square(x=w566) -> (x^2=w576:dbl)
                                n309 = Absolute Value(x=w567) -> (abs(x)=w574:dbl)
                                n310 = Greater Or Equal?(x=w574, y=w566) -> (x >= y?=w573:bool)
                                n311 = Add(x=w575, y=w576) -> (x+y=w577:dbl)
                                n312 = Divide(x=w577, y=w567) -> (x/y=w578:dbl)
                                n313 = Multiply(x=w578, y=0.5) -> (x*y=w580:dbl)
                                n314 = Select(t=w567, s=w573, f=w580) -> (s? t:f=w568:dbl)
                                n315 = Not A Number/Path/Refnum?(number/path/refnum=w568) -> (NaN/Path/Refnum?=w571:bool)
                                n316 = global read "rio_Global.vi" "wheel base"() -> (w572:dbl)
                                n317 = Select(t=inf, s=w571, f=w568) -> (s? t:f=w569:dbl)
                                n318 = Divide(x=w572, y=w569) -> (x/y=w581:dbl)
                                n319 = Inverse Tangent(1:w581) -> (0:w564:dbl)
                                }
                                n320 = Increment(x=w548) -> (x+1=w547:i32[])
                                n321 = Add Array Elements(numeric array=w547) -> (sum=w563:i32)
                                n322 = Divide(x=w547, y=w563) -> (x/y=w561:dbl[])
                                n323 = Multiply(x=w562, y=w561) -> (x*y=w560:dbl[])
                                n324 = Add Array Elements(numeric array=w560) -> (sum=w559:dbl)
                              }
                            }
                            n325 = Multiply(x=180.0 ("y"), y=w521) -> (x*y=w522:dbl)
                            n326 = Divide(x=w522, y=3.141592653589793) -> (x/y=w524:dbl)
                            n327 = global read "rio_Global.vi" "ratio"() -> (w509:dbl)
                            n328 = Multiply(x=w509, y=w524) -> (x*y=w508:dbl)
                            n329 = Multiply(x=w508, y=1.0 ("y 3")) -> (x*y=w507:dbl)
                            n330 = Negate(x=w507) -> (-x=w518:dbl)
                            n331 = local read "handle"() -> (w516:dbl)
                            n332 = Not A Number/Path/Refnum?(number/path/refnum=w518) -> (NaN/Path/Refnum?=w519:bool)
                            n333 = Multiply(x=w516, y="str_gain") -> (x*y=w512:dbl)
                            n334 = Decrement(x="str_gain") -> (x-1=w514:dbl)
                            n335 = Select(t=w516, s=w519, f=w518) -> (s? t:f=w513:dbl)
                            n336 = Multiply(x=w514, y=w513) -> (x*y=w511:dbl)
                            n337 = Subtract(x=w512, y=w511) -> (x-y=w510:dbl)
                          }
                        }
                      }
                      frame True {
                        n338 = local read "handle"() -> (w584:dbl)
                        n339 = Multiply(x=w584, y=0.995) -> (x*y=w583:dbl)
                      }
                    }
                    "handle" <- w405
                    n340 = Negate(x=w405) -> (-x=w403:dbl)
                    n341 = Multiply(x=w403, y="gain") -> (x*y=w402:dbl)
                    n342 = global write "rio_Global.vi" "Ref_str_ang"(w402) -> ()
                  }
                  frame #1 {
                    w591 = 2 ("index")
                    w594 = 2 ("index")
                    n343 = global read "rio_Global.vi" "M_lane_right"() -> (w586:dbl[])
                    n344 = global read "rio_Global.vi" "M_lane_left"() -> (w587:dbl[])
                    n345 = Index Array(array=w587, index=w594) -> (element=w593:dbl)
                    n346 = Index Array(array=w586, index=w591) -> (element=w592:dbl)
                    n347 = Greater Or Equal?(x=w593, y=w594) -> (x >= y?=w588:bool)
                    n348 = Greater Or Equal?(x=w592, y=w591) -> (x >= y?=w589:bool)
                    n349 = Or(x=w588, y=w589) -> (x .or. y?=w590:bool)
                    n350 = case shown="False" w590 {
                      tunnel: w589 -> [_ w622]
                      tunnel: [w595 w611] -> w585
                      tunnel: w588 -> [_ w625]
                      tunnel: w587 -> [_ w616]
                      tunnel: w586 -> [_ w615]
                      frame False {
                        n351 = global read "rio_Global.vi" "Ref_str_torque"() -> (w596:dbl)
                        n352 = Multiply(x=w596, y=0.997) -> (x*y=w595:dbl)
                      }
                      frame True {
                        n353 = disable-structure shown="Enabled" {
                          disable-tunnel: [w630 w633] -> w621
                          disable-tunnel: [w629 w655] -> w619
                          disable-tunnel: w616 -> [w628 w664]
                          disable-tunnel: w615 -> [w627 w634]
                          frame Disabled {
                            n354 = Index Array(array=w628, index=5) -> (element=w629:dbl)
                            n355 = Index Array(array=w627, index=5) -> (element=w630:dbl)
                          }
                          frame Enabled {
                            n356 = global read "rio_Global.vi" "C_VS_CAN"() -> (w663:dbl)
                            n357 = global read "rio_Global.vi" "C_VS_CAN"() -> (w639:dbl)
                            n358 = In Range and Coerce(upper limit=45.0, x=w663, lower limit=15.0) -> (coerced(x)=w652:dbl)  [unwired: 1 out]
                            n359 = In Range and Coerce(upper limit=45.0, x=w639, lower limit=15.0) -> (coerced(x)=w649:dbl)  [unwired: 1 out]
                            n360 = Index Array(array=w664, index #1=7 ("index"), index #2=6 ("index"), index #3=9 ("index"), index #4=5 ("index")) -> (element #1=w660:dbl, element #2=w653:dbl, element #3=w651:dbl, element #4=w656:dbl)
                            n361 = Index Array(array=w634, index #1=7 ("index"), index #2=6 ("index"), index #3=9 ("index"), index #4=5 ("index")) -> (element #1=w642:dbl, element #2=w648:dbl, element #3=w650:dbl, element #4=w646:dbl)
                            n362 = Square(x=w652) -> (x^2=w654:dbl)
                            n363 = Square(x=w649) -> (x^2=w647:dbl)
                            n364 = Multiply(x=w654, y=w653) -> (x*y=w658:dbl)
                            n365 = Multiply(x=w652, y=w651) -> (x*y=w657:dbl)
                            n366 = Multiply(x=w647, y=w648) -> (x*y=w644:dbl)
                            n367 = Multiply(x=w649, y=w650) -> (x*y=w645:dbl)
                            n368 = Compound Arithmetic op=MULTIPLY(w660, w654, w652) -> (w659:dbl)
                            n369 = Compound Arithmetic op=MULTIPLY(w642, w647, w649) -> (w643:dbl)
                            n370 = Compound Arithmetic op=ADD(w659, w658, w657, w656) -> (w655:dbl)
                            n371 = Compound Arithmetic op=ADD(w643, w644, w645, w646) -> (w633:dbl)
                          }
                        }
                        n372 = global read "rio_Global.vi" "C_VS_CAN"() -> (w614:dbl)
                        n373 = Square(x=w614) -> (x^2=w613:dbl)
                        n374 = global read "rio_Global.vi" "lane width"() -> (w618:dbl)
                        n375 = Divide(x=w613, y=-28800.0) -> (x/y=w610:dbl)
                        n376 = Subtract(x=w621, y=w618) -> (x-y=w623:dbl)
                        n377 = Add(x=w619, y=w618) -> (x+y=w617:dbl)
                        n378 = global read "rio_Global.vi" "C_Right light"() -> (w602:bool)
                        n379 = Multiply(x=w610, y="invgain>1") -> (x*y=w609:dbl)
                        n380 = Select(t=w619, s=w625, f=w623) -> (s? t:f=w624:dbl)
                        n381 = Select(t=w621, s=w622, f=w617) -> (s? t:f=w620:dbl)
                        n382 = global read "rio_Global.vi" "C_Left light"() -> (w600:bool)
                        n383 = Negate(x=w624) -> (-x=w626:dbl)
                        n384 = Exponential(1:w609) -> (0:w606:dbl)
                        n385 = Subtract(x=w626, y=w620) -> (x-y=w599:dbl)
                        n386 = Exclusive Or(1:w602, 2:w600) -> (0:w601:bool)
                        n387 = Multiply(x=w606, y=0.125) -> (x*y=w605:dbl)
                        n388 = case shown="True" w601 {
                          tunnel: w600 -> [_ w675]
                          tunnel: [w669 w670] -> w598
                          tunnel: w599 -> [w669 w672]
                          frame False {
                          }
                          frame True {
                            n389 = Select(t=1.0, s=w675, f=-1.0) -> (s? t:f=w671:dbl)
                            n390 = Add(x=w672, y=w671) -> (x+y=w670:dbl)
                          }
                        }
                        n391 = Max & Min(x=w605, y=0.01) -> (max(x,y)=w604:dbl)  [unwired: 1 out]
                        n392 = Multiply(x=w598, y=w604) -> (x*y=w611:dbl)
                      }
                    }
                    n393 = global write "rio_Global.vi" "Ref_str_torque"(w585) -> ()
                  }
                }
              }
              frame "CON_INPUT_T" {
                n394 = global read "rio_Global.vi" "CON_INPUT_T 2"() -> (w678:T26)
                n395 = Unflatten From String(type=w678, binary string=w676, data includes array or string size? (T)=FALSE) -> (value=w677:T26, error out=w679:errorcluster)  [unwired: 2 in, 1 out]
                n396 = case shown="Error" w679 {
                  tunnel: w677 -> [w684 _]
                  tunnel: w676 -> [_ w691]
                  frame No Error {
                    n397 = Unbundle By Name(w684) -> ("ref_vel"=w683:dbl, "ref_steer"=w682:dbl)
                    n398 = global write "rio_Global.vi" "Ref_VS"(w683) -> ()
                    n399 = Negate(x=w682) -> (-x=w681:dbl)
                    n400 = global write "rio_Global.vi" "Ref_str_ang"(w681) -> ()
                  }
                  frame Error {
                    n401 = global read "rio_Global.vi" "CON_INPUT_T"() -> (w689:T27)
                    n402 = Unflatten From String(type=w689, binary string=w691, data includes array or string size? (T)=FALSE) -> (value=w685:T27)  [unwired: 2 in, 2 out]
                    n403 = Unbundle By Name(w685) -> ("ref_vel"=w688:dbl, "ref_steer"=w687:dbl)
                    n404 = Negate(x=w687) -> (-x=w686:dbl)
                    n405 = global write "rio_Global.vi" "Ref_VS"(w688) -> ()
                    n406 = global write "rio_Global.vi" "Ref_str_ang"(w686) -> ()
                  }
                }
              }
            }
          }
          frame #2 {
            n407 = global read "rio_Global.vi" "Ref_VS"() -> (w700:dbl)
            n408 = global read "rio_Global.vi" "C_gear selector disp"() -> (w692:u8)
            "Gear" <- w692
            n409 = Select(t=w700, s="Velocity input", f="manual speed") -> (s? t:f=w696:dbl)
            n410 = Sign(1:w696) -> (0:w695:dbl)
            n411 = To Long Integer(number=w695) -> (32bit integer=w694:i32)
            n412 = case shown="-1" w694 {
              tunnel: [w702 _ w708] -> w693
              tunnel: w692 -> [w705 _ w711]
              frame -1 {
                n413 = Not Equal?(x=w705, y=u8 1) -> (x != y?=w704:bool)
                n414 = Select(t=-2.0 ("element"), s=w704, f=0.0) -> (s? t:f=w702:dbl)
              }
              frame 0, Default {
              }
              frame 1 {
                n415 = Not Equal?(x=w711, y=u8 3) -> (x != y?=w709:bool)
                n416 = Select(t=2.0 ("element"), s=w709, f=0.0) -> (s? t:f=w708:dbl)
              }
            }
            n417 = case shown="1" w692 {
              tunnel: [_ w713 w718] -> w697
              tunnel: w696 -> [_ w715 w719]
              frame 0, Default {
                # "P,N"
              }
              frame 3 {
                # "D"
                n418 = Greater Than 0?(x=w715) -> (x > 0?=w716:bool)
                n419 = Select(t=w715, s=w716, f=0.0) -> (s? t:f=w713:dbl)
              }
              frame 1 {
                # "R"
                n420 = Less Than 0?(x=w719) -> (x < 0?=w720:bool)
                n421 = Select(t=w719, s=w720, f=0.0) -> (s? t:f=w718:dbl)
              }
            }
            n422 = global write "rio_Global.vi" "Shift control"(w693) -> ()
          }
          frame #3 {
            n423 = global read "rio_Global.vi" "C_VS_CAN"() -> (w725:dbl)
            n424 = global read "rio_Global.vi" "C_VS_CAN"() -> (w723:dbl)
            n425 = global read "rio_Global.vi" "C_MCP"() -> (w730:dbl)
            n426 = global read "rio_Global.vi" "C_APV"() -> (→"APV":dbl)
            n427 = feedback #1(w723) -> (w722:dbl)
            n428 = feedback-in #1(w723) -> ()
            n429 = Subtract(x=w721, y=w725) -> (x-y=w724:dbl)
            n430 = Less?(x=w730, y=5.0) -> (x < y?=w729:bool)
            n431 = case shown="True" w729 {
              tunnel: w721 -> [_ w793]
              tunnel: [_ w780] -> w738
              tunnel: w723 -> [_ w779]
              tunnel: w722 -> [_ w778]
              frame False {
              }
              frame True {
                w785 = 0.09999999999999998 ("lpf gain speed")
                n432 = Subtract(x=w779, y=w778) -> (x-y=w789:dbl)
                n433 = Multiply(x=w789, y=5.0) -> (x*y=w788:dbl)
                n434 = Add(x=w779, y=w788) -> (x+y=w787:dbl)
                n435 = Subtract(x=w793, y=w787) -> (x-y=w792:dbl)
                n436 = local read "fake_Ref_speed"() -> (w784:dbl)
                n437 = Decrement(x=w785) -> (x-1=w783:dbl)
                n438 = Multiply(x=45.0 ("x 2"), y=w792) -> (x*y=w786:dbl)
                n439 = Multiply(x=w786, y=w785) -> (x*y=w782:dbl)
                n440 = Multiply(x=w783, y=w784) -> (x*y=w781:dbl)
                n441 = Subtract(x=w782, y=w781) -> (x-y=w780:dbl)
              }
            }
            n442 = Less?(x=w724, y=-2.0 ("lower limit")) -> (x < y?=w727:bool)
            n443 = case shown="True" w727 {
              tunnel: [w745 w767] -> w726
              tunnel: w721 -> [w749 w768]
              tunnel: w724 -> [w751 w759]
              frame False {
                n444 = global read "rio_Global.vi" "PWM Brake"() -> (w758:dbl)
                n445 = Greater?(x=w751, y=1.0) -> (0:w754:bool)
                n446 = Equal To 0?(x=w749) -> (x = 0?=w748:bool)
                n447 = Multiply(x=w758, y=0.999) -> (x*y=w756:dbl)
                n448 = Max & Min(x=w756, y=1000.0) -> (max(x,y)=w752:dbl)  [unwired: 1 out]
                n449 = Select(t=1000.0, s=w754, f=w752) -> (s? t:f=w746:dbl)
                n450 = Select(t=2000.0, s=w748, f=w746) -> (s? t:f=w745:dbl)
              }
              frame True {
                w765 = 0.5 ("gain brake")
                w774 = 10.0 ("y")
                n451 = Absolute Value(x=w759) -> (abs(x)=w776:dbl)
                n452 = Add(x=w776, y=w774) -> (x+y=w775:dbl)
                n453 = Multiply(x=w775, y=w774) -> (x*y=w773:dbl)
                n454 = Threshold 1D Array(2:w773, 3:dbl[] [10.0, 15.0, 25.0, 50.0, 80.0, 120.0, 170.0, 230.0, 290.0, 350.0, 420.0]) -> (0:w771:dbl)  [unwired: 1 in]
                n455 = global read "rio_Global.vi" "PWM Brake"() -> (w763:dbl)
                n456 = Interpolate 1D Array(1:w771, 2:dbl[] [1000.0, 1100.0, 1200.0, 1300.0, 1400.0, 1500.0, 1600.0, 1700.0, 1800.0, 1900.0, 2000.0]) -> (0:w766:dbl)
                n457 = Decrement(x=w765) -> (x-1=w764:dbl)
                n458 = Multiply(x=w766, y=w765) -> (x*y=w761:dbl)
                n459 = Multiply(x=w764, y=w763) -> (x*y=w762:dbl)
                n460 = Subtract(x=w761, y=w762) -> (x-y=w760:dbl)
                n461 = Equal To 0?(x=w768) -> (x = 0?=w769:bool)
                n462 = Select(t=2000.0, s=w769, f=w760) -> (s? t:f=w767:dbl)
              }
            }
            n463 = global read "rio_Global.vi" "C_MCP"() -> (w736:dbl)
            n464 = global read "rio_Global.vi" "Auto"() -> (w733:bool)
            "Auto" <- w733
            n465 = local read "T out"() -> (w740:i32)
            n466 = local read "T init"() -> (w739:i32)
            n467 = Greater Or Equal?(x=w739, y=w740) -> (x >= y?=w734:bool)
            n468 = Less?(x=w736, y=5.0) -> (x < y?=w742:bool)
            n469 = Compound Arithmetic op=AND(w733, w742, w734) -> (w741:bool)
            n470 = local write "fake_Ref_speed"(w738) -> ()
            n471 = case shown="True" w741 {
              tunnel: [1000.0 ("Numeric") w809] -> w732
              tunnel: w738 -> [_ w804]
              tunnel: w740 -> [w794 _]
              tunnel: [_ TRUE] -> w735
              frame False {
                n472 = local read "T init"() -> (w795:i32)
                n473 = Less Or Equal?(x=w795, y=w794) -> (x <= y?=w796:bool)
                n474 = case shown="True" w796 {
                  tunnel: w794 -> [_ w799]
                  frame False {
                    n475 = local write "T init"(1 ("T init")) -> ()
                  }
                  frame True {
                    n476 = local read "T init"() -> (w802:i32)
                    n477 = Increment(x=w802) -> (x+1=w801:i32)
                    n478 = Max & Min(x=w801, y=w799) -> (min(x,y)=w800:i32)  [unwired: 1 out]
                    n479 = local write "T init"(w800) -> ()
                  }
                }
              }
              frame True {
                w808 = 1000.0 ("x")
                n480 = Add(x=w804, y=1000.0 ("PWM GAS")) -> (x+y=w811:dbl)
                n481 = In Range and Coerce(upper limit=1700.0, x=w811, lower limit=w808) -> (coerced(x)=w809:dbl)  [unwired: 1 out]
                n482 = Subtract(x=w809, y=w808) -> (x-y=w807:dbl)
                n483 = Multiply(x=w807, y=0.1) -> (x*y=w805:dbl)
                n484 = To Long Integer(number=w805) -> (32bit integer=w814:i32)
                n485 = Add(x=w814, y=20) -> (x+y=w816:i32)
                "T out" <- w816
                n486 = Increment(x=w816) -> (x+1=→"T init":i32)
              }
            }
            "PWM GAS" <- w732
            n487 = disable-structure shown="Enabled" {
              disable-tunnel: w726 -> [w744 _]
              frame Enabled {
                n488 = global write "rio_Global.vi" "PWM Brake"(w744) -> ()
              }
              frame Disabled {
              }
            }
            n489 = global write "rio_Global.vi" "Solenoid"(w735) -> ()
            n490 = global write "rio_Global.vi" "PWM GAS"(w732) -> ()
            "Ref_VS" <- w721
          }
          frame #4 {
            n491 = disable-structure shown="Disabled" {
              disable-tunnel: [w827 TRUE] -> w825
              frame Disabled {
                n492 = global read "rio_Global.vi" "C_Right light"() -> (w828:bool)
                n493 = global read "rio_Global.vi" "C_Left light"() -> (w829:bool)
                n494 = Not Or(1:w828, 2:w829) -> (0:w827:bool)
              }
              frame Enabled {
              }
            }
            n495 = global read "rio_Global.vi" "C_mdps str_ang"() -> (w826:dbl)
            n496 = And(x="Steering Control", y=w825) -> (x .and. y?=w823:bool)
            n497 = case shown="True" w823 {
              tunnel: [w831 w845] -> w819
              tunnel: w826 -> [_ w867]
              frame False {
                n498 = local write "fake_Ref_str_ang"(0.0 ("Manual Steering angle")) -> ()
                n499 = global read "rio_Global.vi" "steering torque"() -> (w833:dbl)
                n500 = Multiply(x=w833, y=0.9) -> (x*y=w831:dbl)
              }
              frame True {
                n501 = global read "rio_Global.vi" "Ref_str_ang"() -> (w870:dbl)
                n502 = Select(t=w870, s="Steering angle input", f="Steering angle input") -> (s? t:f=w844:dbl)
                n503 = Add(x=w844, y="shift") -> (x+y=w842:dbl)
                n504 = Subtract(x=w842, y=w867) -> (x-y=w852:dbl)
                n505 = global write "rio_Global.vi" "cmd steer"(w842) -> ()
                n506 = disable-structure shown="Enabled" {
                  disable-tunnel: w852 -> [w876 w880]
                  disable-tunnel: [w874 w880] -> w851
                  frame Enabled {
                    n507 = Absolute Value(x=w876) -> (abs(x)=w879:dbl)
                    n508 = Greater?(x=w879, y=0.001) -> (0:w877:bool)
                    n509 = Select(t=w876, s=w877, f=0.0) -> (s? t:f=w874:dbl)
                  }
                  frame Disabled {
                  }
                }
                n510 = Absolute Value(x=w851) -> (abs(x)=w861:dbl)
                n511 = Sign(1:w851) -> (0:w858:dbl)
                n512 = Multiply(x="x 2", y=w861) -> (x*y=w860:dbl)
                n513 = Square Root(x=w860) -> (sqrt(x)=w859:dbl)
                n514 = Multiply(x=w859, y=w858) -> (x*y=w857:dbl)
                n515 = In Range and Coerce(upper limit=0.4, x=w857, lower limit=-0.4) -> (coerced(x)=w862:dbl, In Range?=w863:bool)
                n516 = case shown="True" w863 {
                  tunnel: w851 -> [_ w885]
                  tunnel: [_ w882] -> w854
                  frame False {
                  }
                  frame True {
                    n517 = Sign(1:w885) -> (0:w884:dbl)
                    n518 = local read "fake_Ref_str_ang"() -> (w886:dbl)
                    n519 = Multiply(x=w884, y="y") -> (x*y=w883:dbl)
                    n520 = Add(x=w886, y=w883) -> (x+y=w882:dbl)
                  }
                }
                n521 = disable-structure shown="Enabled" {
                  disable-tunnel: [w871 "Ref_str_torque"] -> w836
                  frame Enabled {
                    n522 = global read "rio_Global.vi" "Ref_str_torque"() -> (w872:dbl)
                    n523 = Negate(x=w872) -> (-x=w871:dbl)
                  }
                  frame Disabled {
                  }
                }
                n524 = In Range and Coerce(upper limit=0.4, x=w854, lower limit=-0.4) -> (coerced(x)=w853:dbl)  [unwired: 1 out]
                n525 = global read "rio_Global.vi" "steering torque"() -> (w850:dbl)
                n526 = In Range and Coerce(upper limit=0.4, x=w836, lower limit=-0.4) -> (coerced(x)=w835:dbl)  [unwired: 1 out]
                n527 = Add(x=w862, y=w853) -> (x+y=w840:dbl)
                n528 = local write "fake_Ref_str_ang"(w853) -> ()
                n529 = Multiply(x=w850, y="lpf") -> (x*y=w846:dbl)
                n530 = Decrement(x="lpf") -> (x-1=w848:dbl)
                n531 = Select(t=w840, s="mode", f=w835) -> (s? t:f=w839:dbl)
                n532 = Multiply(x=w848, y=w839) -> (x*y=w847:dbl)
                n533 = Subtract(x=w846, y=w847) -> (x-y=w845:dbl)
              }
            }
            n534 = Add(x=w819, y=-0.031 ("y 2")) -> (x+y=w818:dbl)
            n535 = global read "rio_Global.vi" "Auto"() -> (w822:bool)
            n536 = Select(t=w818, s=w822, f=0.0) -> (s? t:f=w820:dbl)
            n537 = global write "rio_Global.vi" "steering torque"(w820) -> ()
          }
          frame #5 {
            n538 = global read "rio_Global.vi" "Auto"() -> (w914:bool)
            n539 = Get Date/Time In Seconds() -> (seconds since 1Jan1904=w904:timestamp)
            n540 = global read "rio_Global.vi" "C_mdps str_ang"() -> (→"mdps str_ang":dbl)
            n541 = global read "rio_Global.vi" "steering torque"() -> (w913:dbl)
            n542 = global read "rio_Global.vi" "Ref_str_torque"() -> (w888:dbl)
            n543 = global read "rio_Global.vi" "LCM_CON_T"() -> (w900:T28)
            n544 = To Double Precision Float(number=w904) -> (double precision float=w905:dbl)
            n545 = case shown="False" w914 {
              frame False {
                w918 = 0.0 ("Manual Steering angle")
                n546 = local write "fake_Ref_str_ang"(w918) -> ()
                n547 = local write "fake_Ref_speed"(w918) -> ()
              }
              frame True {
              }
            }
            n548 = Negate(x=w888) -> (-x=w887:dbl)
            n549 = global read "rio_Global.vi" "cmd steer"() -> (w890:dbl)
            n550 = Unbundle By Name(w900) -> ("hash"=w907:i64)
            n551 = Multiply(x=w905, y=1000000.0) -> (x*y=w903:dbl)
            n552 = Build Array(w887, w913) -> (w916:dbl[])
            n553 = global read "rio_Global.vi" "PWM Brake"() -> (w896:dbl)
            n554 = global read "rio_Global.vi" "PWM GAS"() -> (w895:dbl)
            n555 = global read "rio_Global.vi" "Solenoid"() -> (w897:bool)
            n556 = To Quad Integer(1:w903) -> (0:w912:i64)
            n557 = Negate(x=w890) -> (-x=w889:dbl)
            n558 = call "hash.vi"("input"=w907) -> ("output"=w902:i64)  [unwired: 10 in]
            n559 = call "Convert to Dynamic Data"("Array"=w916) -> ("Dynamic Data Type"=→"Waveform Chart":dynamicdata)  [unwired: 3 in]
            n560 = local read "Ref_VS"() -> (w894:dbl)
            n561 = global read "rio_Global.vi" "Auto"() -> (w899:bool)
            n562 = Bundle(cluster=w900, "hash"=w902, "sys time"=w912, "Auto"=w899, "Run"=w899, "Solenoid"=w897, "T lim"=FALSE, "brk_enc"=u8 0, "B PWM"=w896, "T PWM"=w895, "ref_vel"=w894, "ref_bkr_enc"=0.0, "ref_apv"=0.0, "ref_steer"=w889) -> (w909:T28)
            n563 = Flatten To String(anything=w909, prepend array or string size? (T)=FALSE) -> (data string=w911:string)  [unwired: 2 in, 2 out]
            n564 = global read "rio_Global.vi" "LCM"() -> (w910:T9)
            n565 = call "LCM_send.vi"("DATA"=w911, "ID"="CON_T", "LCM"=w910) -> ()  [unwired: 7 in, 2 out]
          }
        }
      }
    }
  }
  n566 = disable-structure shown="Enabled" {
    frame Enabled {
      n567 = flat-sequence {
        tunnel: [dbl[] [0.0, 0.0, 0.0, 0.0, 0.0] ("pos(i)")] -> w919
        tunnel: w919 -> [w934]
        frame #0 {
          w926 = u64 1
          w923 = 0.0 ("dh_hat")
          n568 = local write "GPS init"(FALSE ("get heading")) -> ()
          n569 = call "getecefdcmref.vi"("map name"=T1."KATRI") -> ("XYZ"=w921:dbl[])  [unwired: 10 in, 4 out]
          n570 = local write "ecef ref"(w921) -> ()
          "vgain" <- 1.04 ("initH")
          "vcount" <- w926
          "hbias" <- w923
          "hcount" <- w926
          "heading error" <- w923
          "pos error" <- w923
          "Kalmann init" <- TRUE ("POS init")
          "get map name" <- TRUE
        }
        frame #1 {
          n571 = disable-structure shown="Enabled" {
            disable-tunnel: w934 -> [w1044 _]
            frame Enabled {
              n572 = node-c288(i64 10 ("Period")) -> (w1043:T2)  [unwired: 3 in]
              n573 = timed-loop {
                shift-right: [w1045] -> _
                shift-left: w1044 -> [w1046]
                timing: w1043 -> [_]
                timing-out: [_] -> w1042
                stop <- FALSE stop-if-true
                n574 = node-c288() -> ()  [unwired: 1 in]
                n575 = flat-sequence {
                  tunnel: [w1062] -> w1048
                  tunnel: w1046 -> [w1062]
                  tunnel: w1048 -> [w1065]
                  tunnel: [w1064] -> w1047
                  tunnel: [w1379] -> w1045
                  tunnel: w1047 -> [w1379]
                  frame #0 {
                    n576 = call "Tick Count"() -> ("Tick Count(uSec)"=w1059:u32)
                    n577 = global read "rio_Global.vi" "C_yaw_rate"() -> (w1054:dbl)
                    n578 = global read "rio_Global.vi" "C_VS_CAN"() -> (→"VS_CAN":dbl)
                    n579 = feedback-in #2(w1059) -> ()
                    n580 = feedback #2(w1059) -> (w1060:u32)
                    n581 = Subtract(x=w1059, y=w1060) -> (x-y=w1058:u32)
                    n582 = Subtract(x=w1054, y=0.25) -> (x-y=→"yaw_rate":dbl)
                    n583 = To Double Precision Float(number=w1058) -> (double precision float=w1057:dbl)
                    n584 = Multiply(x=w1057, y=1e-06) -> (x*y=→"dt":dbl)
                  }
                  frame #1 {
                    n585 = flat-sequence {
                      tunnel: w1065 -> [w1108]
                      tunnel: [w1108] -> w1063
                      tunnel: [w1133] -> w1064
                      tunnel: w1063 -> [w1134]
                      frame #0 {
                        n586 = global read "rio_Global.vi" "gps_pos 1"() -> (w1105:dbl[])
                        "pos_gps" <- w1105
                        n587 = global read "rio_Global.vi" "gps_vel 1"() -> (w1092:dbl[])
                        n588 = local read "VS_CAN"() -> (w1071:dbl)
                        n589 = local read "VS_CAN"() -> (w1070:dbl)
                        n590 = local read "VS_CAN"() -> (w1072:dbl)
                        n591 = Equal To 0?(x=w1071) -> (x = 0?=w1073:bool)
                        n592 = Index Array(array=w1105, index #1=0 ("index")) -> (element #1=w1102:dbl, element #2=w1101:dbl, element #3=w1066:dbl)  [unwired: 2 in]
                        n593 = Index Array(array=w1092, index #1=0 ("index"), index #2=1 ("index"), index #3=4 ("index"), index #4=2 ("index")) -> (element #1=w1075:dbl, element #2=w1088:dbl, element #3=w1085:dbl, element #4=w1077:dbl)
                        n594 = Not Equal To 0?(x=w1101) -> (x != 0?=w1098:bool)
                        n595 = Greater Or Equal To 0?(x=w1070) -> (x >= 0?=w1094:bool)
                        n596 = feedback #3(w1102) -> (w1100:dbl)
                        n597 = feedback-in #3(w1102) -> ()
                        n598 = case shown="True" w1073 {
                          frame False {
                          }
                          frame True {
                            w1112 = u64 18446744073709551615
                            n599 = local read "hcount"() -> (w1115:u64)
                            n600 = local read "hbias"() -> (w1118:dbl)
                            n601 = Increment(x=w1115) -> (x+1=w1114:u64)
                            n602 = local read "yaw_rate"() -> (w1109:dbl)
                            n603 = Not Equal?(x=w1115, y=w1112) -> (x != y?=w1113:bool)
                            n604 = Multiply(x=w1118, y=w1115) -> (x*y=w1117:dbl)
                            n605 = Add(x=w1109, y=w1117) -> (x+y=w1116:dbl)
                            n606 = Select(t=w1114, s=w1113, f=w1112) -> (s? t:f=w1111:u64)
                            n607 = Divide(x=w1116, y=w1111) -> (x/y=w1110:dbl)
                            n608 = local write "hcount"(w1111) -> ()
                            n609 = local write "hbias"(w1110) -> ()
                          }
                        }
                        n610 = Absolute Value(x=w1072) -> (abs(x)=w1078:dbl)
                        n611 = call "Convert to Dynamic Data2"("Double"=w1066) -> ("Dynamic Data Type"=→"Waveform Chart 2":dynamicdata)  [unwired: 3 in]
                        n612 = Greater?(x=w1102, y=w1100) -> (0:w1099:bool)
                        n613 = feedback #4(w1075) -> (w1084:dbl)
                        n614 = feedback-in #4(w1075) -> ()
                        n615 = call "angleconv.vi"("deg"=w1085) -> ("rad"=w1076:dbl)  [unwired: 9 in, 1 out]
                        n616 = Divide(x=w1077, y=w1078) -> (x/y=w1107:dbl)
                        n617 = Select(t=0.0, s=w1094, f=3.141592653589793) -> (s? t:f=w1093:dbl)
                        n618 = And(x=w1099, y=w1098) -> (x .and. y?=→"get position":bool)
                        n619 = Greater?(x=w1075, y=w1084) -> (0:w1089:bool)
                        n620 = call "headingoperater.vi"("h1"=w1093, "h2"=w1076) -> ("h2-h1"=→"h_gps":dbl)  [unwired: 8 in, 1 out]
                        n621 = Not Equal To 0?(x=w1088) -> (x != 0?=w1087:bool)
                        n622 = Decrement(x=w1107) -> (x-1=w1081:dbl)
                        n623 = Absolute Value(x=w1081) -> (abs(x)=w1082:dbl)
                        n624 = And(x=w1089, y=w1087) -> (x .and. y?=w1068:bool)
                        "get heading" <- w1068
                        n625 = Greater?(x=w1078, y=15.0) -> (0:w1069:bool)
                        n626 = Less?(x=w1082, y=0.05) -> (x < y?=w1074:bool)
                        n627 = Compound Arithmetic op=AND(w1068, w1074, w1069) -> (w1106:bool)
                        n628 = case shown="True" w1106 {
                          tunnel: w1107 -> [_ w1126]
                          frame False {
                          }
                          frame True {
                            w1120 = u64 18446744073709551615
                            n629 = local read "vcount"() -> (w1123:u64)
                            n630 = local read "vgain"() -> (w1128:dbl)
                            n631 = Increment(x=w1123) -> (x+1=w1122:u64)
                            n632 = Multiply(x=w1128, y=w1123) -> (x*y=w1127:dbl)
                            n633 = Not Equal?(x=w1123, y=w1120) -> (x != y?=w1121:bool)
                            n634 = Add(x=w1126, y=w1127) -> (x+y=w1125:dbl)
                            n635 = Select(t=w1122, s=w1121, f=w1120) -> (s? t:f=w1119:u64)
                            n636 = local write "vcount"(w1119) -> ()
                            n637 = Divide(x=w1125, y=w1119) -> (x/y=w1124:dbl)
                            n638 = local write "vgain"(w1124) -> ()
                          }
                        }
                      }
                      frame #1 {
                        n639 = local read "dt"() -> (w1132:dbl)
                        n640 = In Range and Coerce(upper limit=0.05, x=w1132, lower limit=1e-06 ("y")) -> (In Range?=w1129:bool)  [unwired: 1 out]
                        n641 = case shown="True" w1129 {
                          tunnel: w1134 -> [w1135 w1138]
                          tunnel: [w1135 w1137] -> w1133
                          frame False {
                          }
                          frame True {
                            n642 = flat-sequence {
                              tunnel: w1138 -> [w1178]
                              tunnel: [w1157] -> w1136
                              tunnel: [w1206] -> w1137
                              tunnel: w1136 -> [w1184]
                              frame #0 {
                                n643 = local read "yaw_rate"() -> (w1145:dbl)
                                n644 = local read "hbias"() -> (w1146:dbl)
                                n645 = local read "VS_CAN"() -> (w1149:dbl)
                                n646 = local read "VS_CAN"() -> (w1148:dbl)
                                n647 = Subtract(x=w1145, y=w1146) -> (x-y=w1143:dbl)
                                n648 = local read "vgain"() -> (w1153:dbl)
                                n649 = Equal To 0?(x=w1148) -> (x = 0?=w1144:bool)
                                n650 = Negate(x=w1143) -> (-x=w1140:dbl)
                                n651 = Multiply(x=w1149, y=w1153) -> (x*y=w1152:dbl)
                                n652 = Select(t=0.0, s=w1144, f=w1140) -> (s? t:f=w1142:dbl)
                                n653 = call "angleconv.vi"("deg"=w1142) -> ("rad"=w1150:dbl)  [unwired: 9 in, 1 out]
                                n654 = Divide(x=w1152, y=3.6) -> (x/y=w1151:dbl)
                                n655 = Index Array(array=w1178, index #1=0 ("index"), index #2=3 ("index"), index #3=1 ("index"), index #4=3 ("index")) -> (element #1=w1172:dbl, element #2=w1171:dbl, element #3=w1167:dbl, element #4=w1162:dbl)
                                n656 = local read "dt"() -> (w1175:dbl)
                                n657 = local read "dt"() -> (w1160:dbl)
                                n658 = Multiply(x=w1151, y=w1175) -> (x*y=w1139:dbl)
                                n659 = Multiply(x=w1160, y=w1150) -> (x*y=w1147:dbl)
                                "rt" <- w1147
                                n660 = Cosine(x=w1171) -> (cos(x)=w1176:dbl)
                                n661 = Sine(x=w1171) -> (sin(x)=w1170:dbl)
                                n662 = Multiply(x=w1176, y=w1139) -> (x*y=w1173:dbl)
                                n663 = Multiply(x=w1139, y=w1170) -> (x*y=w1169:dbl)
                                n664 = Add(x=w1172, y=w1173) -> (x+y=w1166:dbl)
                                n665 = Add(x=w1169, y=w1167) -> (x+y=w1165:dbl)
                                n666 = call "headingoperater.vi"("h1"=w1147, "h2"=w1162) -> ("h2+h1"=w1161:dbl)  [unwired: 8 in, 1 out]
                                n667 = Build Array(w1166, w1165, w1151, w1161, w1150) -> (w1157:dbl[])
                                n668 = Index Array(array=w1157, index=3) -> (element=w1156:dbl)
                                n669 = local read "h_gps"() -> (w1155:dbl)
                                n670 = call "headingoperater.vi"("h1"=w1156, "h2"=w1155) -> ("h2-h1"=w1159:dbl)  [unwired: 8 in, 1 out]
                                n671 = Absolute Value(x=w1159) -> (abs(x)=w1154:dbl)
                                n672 = local write "heading error"(w1154) -> ()
                              }
                              frame #1 {
                                n673 = Array Subset(array=w1184, index=0, length=2) -> (w1191:dbl[])
                                n674 = local read "pos_gps"() -> (w1187:dbl[])
                                n675 = local read "Kalmann init"() -> (w1199:bool)
                                n676 = local read "get heading"() -> (w1212:bool)
                                n677 = local read "get position"() -> (w1211:bool)
                                n678 = Array Subset(array=w1187, index=2, length=2) -> (w1190:dbl[])
                                n679 = Subtract(x=w1190, y=w1191) -> (x-y=w1192:dbl[])
                                n680 = case shown="True" w1199 {
                                tunnel: w1212 -> [w1215 w1222]
                                tunnel: w1211 -> [w1219 w1221]
                                tunnel: [w1213 w1220] -> w1208
                                frame False {
                                n681 = local read "heading error"() -> (w1216:dbl)
                                n682 = Less?(x=w1216, y=0.05) -> (x < y?=w1217:bool)
                                n683 = And(x=w1215, y=w1217) -> (x .and. y?=w1214:bool)
                                n684 = Or(x=w1214, y=w1219) -> (x .or. y?=w1213:bool)
                                }
                                frame True {
                                n685 = disable-structure shown="Enabled" {
                                disable-tunnel: w1222 -> [w1225 w1227]
                                disable-tunnel: w1221 -> [w1224 w1226]
                                disable-tunnel: [w1223 w1228] -> w1220
                                frame Disabled {
                                n686 = And(x=w1225, y=w1224) -> (x .and. y?=w1223:bool)
                                }
                                frame Enabled {
                                n687 = Or(x=w1227, y=w1226) -> (x .or. y?=w1228:bool)
                                }
                                }
                                }
                                }
                                n688 = Square(x=w1192) -> (x^2=w1193:dbl[])
                                n689 = Add Array Elements(numeric array=w1193) -> (sum=w1194:dbl)
                                n690 = Square Root(x=w1194) -> (sqrt(x)=w1183:dbl)
                                n691 = local read "VS_CAN"() -> (w1195:dbl)
                                n692 = local read "heading error"() -> (w1202:dbl)
                                n693 = local read "Kalmann init"() -> (w1200:bool)
                                n694 = Absolute Value(x=w1195) -> (abs(x)=w1210:dbl)
                                n695 = Greater?(x=w1210, y=5.0) -> (0:w1207:bool)
                                n696 = Less?(x=w1202, y=1.0) -> (x < y?=w1201:bool)
                                n697 = Or(x=w1201, y=w1200) -> (x .or. y?=w1203:bool)
                                n698 = And(x=w1208, y=w1207) -> (x .and. y?=w1204:bool)
                                n699 = And(x=w1204, y=w1203) -> (x .and. y?=w1197:bool)
                                n700 = Less?(x=w1183, y=50.0) -> (x < y?=w1180:bool)
                                n701 = Select(t=FALSE, s="GPS init", f=w1197) -> (s? t:f=w1181:bool)
                                n702 = And(x=w1181, y=w1180) -> (x .and. y?=w1179:bool)
                                n703 = case shown="True" w1179 {
                                tunnel: [w1234 w1261] -> w1206
                                tunnel: w1184 -> [w1229 w1264]
                                frame False {
                                n704 = local read "VS_CAN"() -> (w1230:dbl)
                                n705 = local read "Kalmann init"() -> (w1236:bool)
                                n706 = Equal To 0?(x=w1230) -> (x = 0?=w1235:bool)
                                n707 = local read "GPS init"() -> (w1231:bool)
                                n708 = And(x=w1236, y=w1235) -> (x .and. y?=w1233:bool)
                                n709 = Or(x=w1233, y=w1231) -> (x .or. y?=w1232:bool)
                                n710 = case shown="False" w1232 {
                                tunnel: w1229 -> [w1237 w1238]
                                tunnel: [w1237 w1240] -> w1234
                                tunnel: w1231 -> [_ w1239]
                                frame False {
                                }
                                frame True {
                                n711 = case shown="True" w1239 {
                                tunnel: [w1251 w1260] -> w1240
                                tunnel: w1238 -> [w1246 w1254]
                                frame True {
                                n712 = Index Array(array=w1246, index #1=2 ("index")) -> (element #2=w1241:dbl, element #3=w1244:dbl)  [unwired: 2 in, 1 out]
                                n713 = local read "pos_gps"() -> (w1247:dbl[])
                                n714 = local write "GPS init"(FALSE ("GPS init")) -> ()
                                n715 = Index Array(array=w1247, index #1=2 ("index")) -> (element #1=w1249:dbl, element #2=w1248:dbl)  [unwired: 1 in]
                                n716 = local read "h_gps"() -> (w1242:dbl)
                                n717 = Build Array(w1249, w1248, w1241, w1242, w1244) -> (w1251:dbl[])
                                }
                                frame False {
                                w1253 = 0.0 ("element")
                                n718 = Index Array(array=w1254, index=3) -> (element=w1252:dbl)
                                n719 = local read "pos_gps"() -> (w1256:dbl[])
                                n720 = Index Array(array=w1256, index #1=2 ("index")) -> (element #1=w1258:dbl, element #2=w1257:dbl)  [unwired: 1 in]
                                n721 = Build Array(w1258, w1257, w1253, w1252, w1253) -> (w1260:dbl[])
                                }
                                }
                                }
                                }
                                }
                                frame True {
                                n722 = flat-sequence {
                                tunnel: w1264 -> [w1265]
                                tunnel: [w1265] -> w1263
                                tunnel: w1263 -> [w1306]
                                tunnel: [w1306] -> w1262
                                tunnel: w1262 -> [w1350]
                                tunnel: [w1353] -> w1261
                                frame #0 {
                                w1274 = 0.0 ("element")
                                w1278 = 0.0 ("element")
                                w1280 = 0.0 ("element")
                                w1282 = 0.0 ("element")
                                w1284 = 0.0 ("element")
                                n723 = Index Array(array=w1265, index #1=3 ("index"), index #2=2 ("index"), index #3=3 ("index"), index #4=2 ("index")) -> (element #1=w1294:dbl, element #2=w1296:dbl, element #3=w1299:dbl, element #4=w1288:dbl)
                                n724 = Negate(x=w1296) -> (-x=w1295:dbl)
                                n725 = Sine & Cosine(0:w1299) -> (1:w1291:dbl, 2:w1289:dbl)
                                n726 = Multiply(x=w1295, y=w1291) -> (x*y=w1292:dbl)
                                n727 = Multiply(x=w1289, y=w1288) -> (x*y=w1287:dbl)
                                n728 = Cosine(x=w1294) -> (cos(x)=w1293:dbl)
                                n729 = Build Array(w1284, w1284, w1293, w1292, 0.0 ("element")) -> (w1286:dbl[])
                                n730 = Build Array(w1282, w1282, w1291, w1287, 0.0 ("element")) -> (w1285:dbl[])
                                n731 = Build Array(w1280, w1280, w1280, w1280, w1280) -> (w1279:dbl[])
                                n732 = Build Array(w1278, w1278, w1278, w1278, 1.0 ("element")) -> (w1276:dbl[])
                                n733 = Build Array(w1274, w1274, w1274, w1274, w1274) -> (w1275:dbl[])
                                n734 = Build Array(w1286, w1285, w1279, w1276, w1275) -> (w1272:dbl[][])
                                n735 = call-poly <vilib>:"Array To Matrix.vi"("Real 2D Array"=w1272) -> ("Real Matrix"=w1270:T29)
                                n736 = global read "rio_Global.vi" "P"() -> (w1273:T29)
                                n737 = Transpose Matrix(1:w1270) -> (0:w1269:T29)
                                n738 = call-poly <vilib>:"Multiply.vi"("Real Matrix B"=w1273, "Real Matrix A"=w1270) -> ("A * B"=w1271:T29)
                                n739 = call-poly <vilib>:"Multiply.vi"("Real Matrix B"=w1269, "Real Matrix A"=w1271) -> ("A * B"=w1268:T29)
                                n740 = global read "rio_Global.vi" "Q"() -> (w1267:T29)
                                n741 = call-poly <vilib>:"Add.vi"("Real Matrix B"=w1267, "Real Matrix A"=w1268) -> ("A + B"=w1266:T29)
                                n742 = global write "rio_Global.vi" "Pp"(w1266) -> ()
                                }
                                frame #1 {
                                n743 = global read "rio_Global.vi" "Pp"() -> (w1331:T29)
                                n744 = global read "rio_Global.vi" "H"() -> (w1330:T29)
                                n745 = Array Subset(array=w1306, index=0, length=2) -> (w1313:dbl[])
                                n746 = local read "pos_gps"() -> (w1309:dbl[])
                                n747 = call-poly <vilib>:"Multiply.vi"("Real Matrix B"=w1331, "Real Matrix A"=w1330) -> ("A * B"=w1329:T29)
                                n748 = Transpose Matrix(1:w1330) -> (0:w1328:T29)
                                n749 = call-poly <vilib>:"Multiply.vi"("Real Matrix B"=w1328, "Real Matrix A"=w1329) -> ("A * B"=w1327:T29)
                                n750 = Array Subset(array=w1309, index=2, length=2) -> (w1312:dbl[])
                                n751 = Subtract(x=w1312, y=w1313) -> (x-y=w1314:dbl[])
                                n752 = global read "rio_Global.vi" "H"() -> (w1325:T29)
                                n753 = global read "rio_Global.vi" "R"() -> (w1326:T29)
                                n754 = global read "rio_Global.vi" "Pp"() -> (w1324:T29)
                                n755 = call-poly <vilib>:"Add.vi"("Real Matrix B"=w1326, "Real Matrix A"=w1327) -> ("A + B"=w1321:T29)
                                n756 = Square(x=w1314) -> (x^2=w1315:dbl[])
                                n757 = Transpose Matrix(1:w1325) -> (0:w1323:T29)
                                n758 = local read "heading error"() -> (w1318:dbl)
                                n759 = call-poly <vilib>:"Multiply.vi"("Real Matrix B"=w1323, "Real Matrix A"=w1324) -> ("A * B"=w1322:T29)
                                n760 = Add Array Elements(numeric array=w1315) -> (sum=w1316:dbl)
                                n761 = call-poly <vilib>:"Inverse Matrix.vi"("Input Matrix"=w1321) -> ("Inverse Matrix"=w1320:T29)  [unwired: 1 in, 1 out]
                                n762 = call-poly <vilib>:"Multiply.vi"("Real Matrix B"=w1320, "Real Matrix A"=w1322) -> ("A * B"=w1319:T29)
                                n763 = Square Root(x=w1316) -> (sqrt(x)=w1301:dbl)
                                n764 = global write "rio_Global.vi" "K"(w1319) -> ()
                                n765 = local write "pos error"(w1301) -> ()
                                n766 = Less?(x=w1301, y=2.5) -> (x < y?=w1303:bool)
                                n767 = Less?(x=w1318, y=0.05) -> (x < y?=w1304:bool)
                                n768 = And(x=w1304, y=w1303) -> (x .and. y?=w1302:bool)
                                n769 = case shown="True" w1302 {
                                frame False {
                                }
                                frame True {
                                n770 = local write "Kalmann init"(FALSE ("Kalman init")) -> ()
                                }
                                }
                                }
                                frame #2 {
                                n771 = disable-structure shown="Enabled" {
                                disable-tunnel: [w1365 w1366] -> w1352
                                frame Disabled {
                                n772 = local read "get heading"() -> (w1365:bool)
                                }
                                frame Enabled {
                                n773 = local read "heading error"() -> (w1369:dbl)
                                n774 = local read "Kalmann init"() -> (w1367:bool)
                                n775 = Less?(x=w1369, y=0.1) -> (x < y?=w1368:bool)
                                n776 = Or(x=w1368, y=w1367) -> (x .or. y?=w1366:bool)
                                }
                                }
                                n777 = Index Array(array=w1350, index=3) -> (element=w1356:dbl)
                                n778 = global read "rio_Global.vi" "K"() -> (w1364:T29)
                                n779 = global read "rio_Global.vi" "H"() -> (w1363:T29)
                                n780 = global read "rio_Global.vi" "Pp"() -> (w1361:T29)
                                n781 = call-poly <vilib>:"Multiply.vi"("Real Matrix B"=w1363, "Real Matrix A"=w1364) -> ("A * B"=w1362:T29)
                                n782 = global read "rio_Global.vi" "Pp"() -> (w1359:T29)
                                n783 = call-poly <vilib>:"Multiply.vi"("Real Matrix B"=w1361, "Real Matrix A"=w1362) -> ("A * B"=w1360:T29)
                                n784 = call-poly <vilib>:"Subtract.vi"("Real Matrix B"=w1360, "Real Matrix A"=w1359) -> ("A - B"=w1358:T29)
                                n785 = global write "rio_Global.vi" "P"(w1358) -> ()
                                n786 = case shown="True" w1352 {
                                tunnel: w1356 -> [w1371 w1378]
                                tunnel: [w1371 w1373] -> w1351
                                frame False {
                                }
                                frame True {
                                n787 = global read "rio_Global.vi" "K"() -> (w1377:T29)
                                n788 = Index Array(array=w1377, index (row)=3, index (col)=2 ("disabled index (col)")) -> (element=w1374:dbl)
                                n789 = local read "h_gps"() -> (w1372:dbl)
                                n790 = call "headingweightsum2.vi"("a"=w1374, "h2"=w1372, "h1"=w1378) -> ("a*h2+(1-a)*h1"=w1373:dbl)  [unwired: 8 in]
                                }
                                }
                                n791 = local read "pos_gps"() -> (w1336:dbl[])
                                n792 = call-poly <vilib>:"Array To Matrix.vi"("Real 1D Array"=w1350) -> ("Real Matrix (Column Vector)"=w1344:T29)
                                n793 = Array Subset(array=w1336, index=2, length=2) -> (w1337:dbl[])
                                n794 = Build Array (concatenate)(w1337, w1351) -> (w1333:dbl[])
                                n795 = global read "rio_Global.vi" "H"() -> (w1349:T29)
                                n796 = call-poly <vilib>:"Multiply.vi"("Real Matrix B"=w1344, "Real Matrix A"=w1349) -> ("A * B"=w1348:T29)
                                n797 = call-poly <vilib>:"Array To Matrix.vi"("Real 1D Array"=w1333) -> ("Real Matrix (Column Vector)"=w1347:T29)
                                n798 = call-poly <vilib>:"Subtract.vi"("Real Matrix B"=w1348, "Real Matrix A"=w1347) -> ("A - B"=w1345:T29)
                                n799 = global read "rio_Global.vi" "K"() -> (w1346:T29)
                                n800 = call-poly <vilib>:"Multiply.vi"("Real Matrix B"=w1345, "Real Matrix A"=w1346) -> ("A * B"=w1340:T29)
                                n801 = call-poly <vilib>:"Multiply.vi"("Real Matrix A"=w1340, "Real Scalar c"=0.7) -> ("c * A"=w1338:T29)
                                n802 = call-poly <vilib>:"Add.vi"("Real Matrix B"=w1344, "Real Matrix A"=w1338) -> ("A + B"=w1343:T29)
                                n803 = call-poly <vilib>:"Matrix To Array.vi"("Real Matrix"=w1343) -> ("Real 2D Array"=w1342:dbl[][])
                                n804 = Index Array(array=w1342, index (col)=0 ("disabled index (col)")) -> (element=w1355:dbl[])  [unwired: 1 in]
                                n805 = Replace Array Subset(array=w1355, new element=w1351, index=3) -> (w1353:dbl[])
                                }
                                }
                                }
                                }
                              }
                            }
                          }
                        }
                      }
                    }
                  }
                  frame #2 {
                    n806 = local read "h_gps"() -> (w1385:dbl)
                    n807 = local read "dt"() -> (w1382:dbl)
                    n808 = Index Array(array=w1379, index=3) -> (element=w1389:dbl)
                    n809 = Array Subset(array=w1379, index=0, length=2) -> (→"pos":dbl[])
                    n810 = Greater Than 0?(x=w1382) -> (x > 0?=w1381:bool)
                    n811 = call "angleconv.vi"("rad"=w1389) -> ("deg"=→"Heading":dbl)  [unwired: 9 in, 1 out]
                    n812 = Greater?(x=1.0, y=w1382) -> (0:w1384:bool)
                    n813 = call "headingoperater.vi"("h1"=0.0, "h2"=w1385) -> ("h2+h1"=w1386:dbl)  [unwired: 8 in, 1 out]
                    n814 = call "angleconv.vi"("rad"=w1386) -> ("deg"=→"H_GPS":dbl)  [unwired: 9 in, 1 out]
                    n815 = Compound Arithmetic op=AND(w1384, w1381) -> (w1380:bool)
                    n816 = case shown="True" w1380 {
                      tunnel: w1379 -> [_ w1395]
                      frame False {
                      }
                      frame True {
                        n817 = flat-sequence {
                          tunnel: w1395 -> [w1419]
                          frame #0 {
                            n818 = Get Date/Time In Seconds() -> (seconds since 1Jan1904=w1410:timestamp)
                            n819 = To Double Precision Float(number=w1410) -> (double precision float=w1404:dbl)
                            n820 = global read "rio_Global.vi" "LCM_POS_T"() -> (w1418:T30)
                            n821 = local read "Kalmann init"() -> (w1400:bool)
                            n822 = Unbundle By Name(w1418) -> ("hash"=w1415:i64)
                            n823 = local read "dt"() -> (w1399:dbl)
                            n824 = Multiply(x=w1404, y=1000000.0) -> (x*y=w1402:dbl)
                            n825 = Array To Cluster(array=w1419) -> (cluster=w1417:T31)
                            n826 = Select(t=0.0, s=w1400, f=w1399) -> (s? t:f=w1397:dbl)
                            n827 = call "hash.vi"("input"=w1415) -> ("output"=w1414:i64)  [unwired: 10 in]
                            n828 = To Quad Integer(1:w1402) -> (0:w1401:i64)
                            n829 = Unbundle(w1417) -> ("Real 2D Array[0]"=w1409:dbl, "Real 2D Array[1]"=w1408:dbl, "Real 2D Array[2]"=w1407:dbl, "Real 2D Array[3]"=w1406:dbl, "Real 2D Array[4]"=w1405:dbl)
                            n830 = Bundle(cluster=w1418, "hash"=w1414, "sys time"=w1401, "dt"=w1397, "x"=w1409, "y"=w1408, "speed"=w1407, "heading"=w1406, "yaw_rate"=w1405) -> (w1396:T30)
                            n831 = Flatten To String(anything=w1396, prepend array or string size? (T)=FALSE) -> (data string=w1412:string)  [unwired: 2 in, 2 out]
                            n832 = global read "rio_Global.vi" "LCM"() -> (w1411:T9)
                            n833 = call "LCM_send.vi"("DATA"=w1412, "ID"="POS_T", "LCM"=w1411) -> ()  [unwired: 7 in, 2 out]
                          }
                        }
                      }
                    }
                  }
                }
                n834 = node-c288() -> ()  [unwired: 1 in, 1 out]
              }
              n835 = node-c288(w1042) -> ()  [unwired: 1 out]
            }
            frame Disabled {
            }
          }
          n836 = while {
            shift-right: [w1039] -> w930
            shift-left: refnum<visa-resource-name> "ASRL3::INSTR" ("VISA resource name") -> [w1040]
            stop <- w1038 continue-if-true
            n837 = VISA Open(VISA resource name=w1040) -> (VISA resource name=w1039:refnum<visa-resource-name>, error out=w1038:errorcluster)  [unwired: 4 in]
          }
          n838 = VISA Clear(VISA resource name=w930) -> (VISA resource name out=w932:refnum<visa-resource-name>)  [unwired: 1 in, 1 out]
          n839 = property class="Instr"(reference=w932, "General Settings:Timeout Value"=u32 10) -> (reference out=w933:refnum<visa-resource-name>)  [unwired: 1 in, 1 out]
          n840 = while {
            tunnel: w933 -> [w937]
            stop <- FALSE stop-if-true
            n841 = property class="Instr"(reference=w937) -> (reference out=w936:refnum<visa-resource-name>, "Bytes at Port"=w935:u32)  [unwired: 1 in, 1 out]
            n842 = case shown="1, Default" w935 {
              selector: w935 -> [_ w943]
              tunnel: w936 -> [_ w944]
              frame 0 {
                n843 = Wait (ms)(milliseconds to wait=u32 10) -> ()  [unwired: 1 out]
              }
              frame 1, Default {
                n844 = VISA Read(VISA resource name=w944, byte count=w943) -> (read buffer=w945:string)  [unwired: 1 in, 3 out]
                "read buffer" <- w945
                n845 = local read "ecef ref"() -> (w940:dbl[])
                n846 = call "nmea.vi"("ecef ref"=w940, "NMEA"=w945) -> ("output"=w942:dbl[], "type"=w941:u32)  [unwired: 8 in]
                n847 = case shown="1" w941 {
                  tunnel: w942 -> [_ w951 w1013]
                  frame 0, Default {
                  }
                  frame 1 {
                    n848 = Index Array(array=w951, index=1) -> (element=w949:dbl)
                    n849 = Not Equal To 0?(x=w949) -> (x != 0?=w948:bool)
                    n850 = local read "get map name"() -> (w947:bool)
                    n851 = And(x=w948, y=w947) -> (x .and. y?=w946:bool)
                    n852 = case shown="True" w946 {
                      tunnel: w951 -> [w952 w1009]
                      frame False {
                        n853 = global write "rio_Global.vi" "gps_pos 1"(w952) -> ()
                        n854 = disable-structure shown="Enabled" {
                          disable-tunnel: w952 -> [w954 _]
                          frame Enabled {
                            n855 = Index Array(array=w954, index=1) -> (element=w956:dbl)
                            n856 = Not Equal To 0?(x=w956) -> (x != 0?=w953:bool)
                            n857 = case shown="True" w953 {
                              tunnel: w954 -> [_ w976]
                              frame False {
                              }
                              frame True {
                                n858 = Get Date/Time In Seconds() -> (seconds since 1Jan1904=w961:timestamp)
                                n859 = To Double Precision Float(number=w961) -> (double precision float=w960:dbl)
                                n860 = global read "rio_Global.vi" "LCM_GGA_T"() -> (w985:T32)
                                n861 = Array To Cluster(array=w976) -> (cluster=w984:T33)
                                n862 = Unbundle By Name(w985) -> ("hash"=w981:i64)
                                n863 = Multiply(x=w960, y=1000000.0) -> (x*y=w958:dbl)
                                n864 = Unbundle(w984) -> ("output[0]"=w986:dbl, "output[2]"=w975:dbl, "output[3]"=w974:dbl, "output[4]"=w973:dbl, "output[6]"=w972:dbl, "output[7]"=w970:dbl, "output[8]"=w968:dbl, "output[9]"=w966:dbl, "output[12]"=w965:dbl, "output[13]"=w964:dbl, "output[14]"=w963:dbl)  [unwired: 4 out]
                                n865 = local read "map name"() -> (w962:T1)
                                n866 = call "hash.vi"("input"=w981) -> ("output"=w980:i64)  [unwired: 10 in]
                                n867 = To Quad Integer(1:w958) -> (0:w957:i64)
                                n868 = To Long Integer(number=w972) -> (32bit integer=w971:i32)
                                n869 = To Long Integer(number=w970) -> (32bit integer=w969:i32)
                                n870 = To Long Integer(number=w968) -> (32bit integer=w967:i32)
                                n871 = Bundle(cluster=w985, "hash"=w980, "sys time"=w957, "time"=w986, "x"=w975, "y"=w974, "h"=w973, "numSV"=w971, "postype"=w969, "lag"=w967, "hordev"=w966, "lat"=w965, "lon"=w964, "hgt"=w963, "map_idx"=w962) -> (w982:T32)
                                n872 = Flatten To String(anything=w982, prepend array or string size? (T)=FALSE) -> (data string=w978:string)  [unwired: 2 in, 2 out]
                                n873 = global read "rio_Global.vi" "LCM"() -> (w977:T9)
                                n874 = call "LCM_send.vi"("DATA"=w978, "ID"="GGA_1", "LCM"=w977) -> ()  [unwired: 7 in, 2 out]
                              }
                            }
                          }
                          frame Disabled {
                          }
                        }
                      }
                      frame True {
                        n875 = local write "get map name"(FALSE ("get map name")) -> ()
                        n876 = Index Array(array=w1009, index #1=12 ("index")) -> (element #1=w1004:dbl, element #2=w1000:dbl)  [unwired: 1 in]
                        n877 = for {
                          N: 11 -> [_]
                          tunnel: [w1011] -> w998 mode=indexing
                          tunnel: [w1010] -> w996 mode=indexing
                          i -> [w1012]
                          n878 = call "getecefdcmref.vi"("map name"=w1012) -> ("lat"=w1011:dbl, "lon"=w1010:dbl)  [unwired: 10 in, 3 out]
                        }
                        n879 = Multiply(x=w1004, y=3.141592653589793) -> (x*y=w1006:dbl)
                        n880 = Multiply(x=w1000, y=3.141592653589793) -> (x*y=w1002:dbl)
                        n881 = Divide(x=w1006, y=180.0) -> (x/y=w997:dbl)
                        n882 = Divide(x=w1002, y=180.0) -> (x/y=w995:dbl)
                        n883 = Subtract(x=w998, y=w997) -> (x-y=w994:dbl[])
                        n884 = Subtract(x=w996, y=w995) -> (x-y=w993:dbl[])
                        n885 = Square(x=w994) -> (x^2=w992:dbl[])
                        n886 = Square(x=w993) -> (x^2=w991:dbl[])
                        n887 = Add(x=w992, y=w991) -> (x+y=w990:dbl[])
                        n888 = Array Max & Min(array=w990) -> (min index (indices)=w989:i32)  [unwired: 3 out]
                        "map name" <- w989
                        n889 = call "getecefdcmref.vi"("map name"=w989) -> ("XYZ"=→"ecef ref":dbl[])  [unwired: 10 in, 4 out]
                      }
                    }
                  }
                  frame 2 {
                    n890 = global write "rio_Global.vi" "gps_vel 1"(w1013) -> ()
                    n891 = disable-structure shown="Enabled" {
                      disable-tunnel: w1013 -> [w1017 _]
                      frame Enabled {
                        n892 = Index Array(array=w1017, index=1) -> (element=w1016:dbl)
                        n893 = Not Equal To 0?(x=w1016) -> (x != 0?=w1014:bool)
                        n894 = case shown="True" w1014 {
                          tunnel: w1017 -> [_ w1036]
                          frame False {
                          }
                          frame True {
                            n895 = Get Date/Time In Seconds() -> (seconds since 1Jan1904=w1022:timestamp)
                            n896 = To Double Precision Float(number=w1022) -> (double precision float=w1021:dbl)
                            n897 = global read "rio_Global.vi" "LCM_RMC_T"() -> (w1037:T34)
                            n898 = Unbundle By Name(w1037) -> ("hash"=w1033:i64)
                            n899 = Multiply(x=w1021, y=1000000.0) -> (x*y=w1019:dbl)
                            n900 = Array To Cluster(array=w1036) -> (cluster=w1035:T35)
                            n901 = To Quad Integer(1:w1019) -> (0:w1018:i64)
                            n902 = call "hash.vi"("input"=w1033) -> ("output"=w1032:i64)  [unwired: 10 in]
                            n903 = Unbundle(w1035) -> ("output[0]"=w1027:dbl, "output[2]"=w1026:dbl, "output[4]"=w1025:dbl, "output[5]"=w1024:dbl, "output[6]"=w1023:dbl)  [unwired: 2 out]
                            n904 = Bundle(cluster=w1037, "hash"=w1032, "sys time"=w1018, "time"=w1027, "speed"=w1026, "heading"=w1025, "lat"=w1024, "lon"=w1023) -> (w1028:T34)
                            n905 = Flatten To String(anything=w1028, prepend array or string size? (T)=FALSE) -> (data string=w1030:string)  [unwired: 2 in, 2 out]
                            n906 = global read "rio_Global.vi" "LCM"() -> (w1029:T9)
                            n907 = call "LCM_send.vi"("DATA"=w1030, "ID"="RMC_1", "LCM"=w1029) -> ()  [unwired: 7 in, 2 out]
                          }
                        }
                      }
                      frame Disabled {
                      }
                    }
                  }
                }
              }
            }
          }
        }
      }
    }
    frame Disabled {
    }
  }
  n908 = flat-sequence {
    tunnel: [w1424] -> w1
    tunnel: w1 -> [w1431]
    frame #0 {
      n909 = for {
        N: 257 -> [_]
        tunnel: [w1430] -> w1428 mode=indexing
        i -> [w1430]
      }
      n910 = Multiply(x=w1428, y=0.5) -> (x*y=w1424:dbl[])
      n911 = global write "rio_Global.vi" "x_view 2"(w1424) -> ()
      n912 = Array Subset(array=w1424, index=30) -> (w1425:dbl[])  [unwired: 1 in]
      n913 = global write "rio_Global.vi" "x_view"(w1425) -> ()
    }
    frame #1 {
      n914 = while {
        tunnel: w1431 -> [w1432]
        stop <- FALSE stop-if-true
        n915 = flat-sequence {
          tunnel: [w1435] -> w1433
          tunnel: w1432 -> [w1435]
          tunnel: w1433 -> [w1437]
          frame #0 {
            n916 = Wait Until Next ms Multiple(millisecond multiple=u32 33) -> ()  [unwired: 1 out]
          }
          frame #1 {
            n917 = call "mobileye_disp.vi"("x_view"=w1437) -> ("XY Graph"=→"XY Graph":cluster{"Y":dbl[], "Y":dbl[]}[])  [unwired: 10 in]
          }
        }
      }
    }
  }
